vi "#SPI_TOF_LIDAR_cz_yuanshi.vi"() -> ()   [LabVIEW 2020]
uses:
  Control 1_.ctl
  Control 2_.ctl
  <vilib>/Analysis/baseanly.llb/Mean (DBL).vi
  handle_ALP_error.vi
  <vilib>/Utility/error.llb/Error Cluster From Error Code.vi
  <vilib>/Analysis/NI_AALBase.lvlib
  <vilib>/gmath/NI_Gmath.lvlib
panel:
  out "Rapid Block Acquisition Settings":T1={"preTriggerSamples"=0, "postTriggerSamples"=1000, "timebase"=2, "Four Channel Device"=FALSE, "Oversample"=1, "Number of Captures"=1}
  in  "index (row)":i32
  out "数组":i16[](array[numeric])
  in  "y 2":dbl
  in  "Tab Control 2":T2(tab)
  out "Resolution":i32=32 min=16 max=128 step=16
  in  "Max Resolution":enum16{"128", "64", "32", "16"}(ring)=enum."32"
  in  "Pulses/Pattern":i32=4
  in  "ms to wait":u32
  in  "Trigger Settings":T3={"Trigger Enabled"=TRUE, "Trigger Source"=enum."Channel C", "Trigger Threshold"=10, "Trigger Direction"=2, "Trigger Delay (samples)"=40, "Auto Trigger Time (ms)"=1000} {"Trigger Direction" items=["Rising"=2, "Falling"=3]}
  out "Captures":u32=10240
  in  "Post Trig. Samples":u32=30
  out "Patterns Loaded":dbl(slide)=2048.0 scale=0.0..2048.0
  in  "Initialised?":bool
  in  "y":dbl=0.9
  out "picture time s":dbl=0.0005142857142857143 format="%#.3p"
  out "1/x":dbl=0.00014285714285714287 format="%#.3p"
  in  "Pre Trigger Samples":u32
  in  "DMD Mode":enum16{"Slave - LUT", "Slave - All Patterns"}(ring)
  in  "Patterns to display":u32(slide)=1024 min=1 max=4096 step=1 scale=0.0..1024.0
  in  "Adaptive Slider":dbl(slide)=1.0 min=0.0 max=1.0 step=0.01 scale=0.0..1.0
  in  "Evolutionary":bool
  in  "Patterns":enum16{"Hadamard", "Random", "Democratised"}(ring)
  in  "learned":bool
  in  "Additional Data":dbl=1.25 format="%#_13g"
  in  "Smooth (pixels)":dbl=0.4 format="%#_13g"
  in  "ntimes":i32=4
  in  "Thresholded":bool
  in  "First":bool
  in  "upsample factor":i32=1
  in  "Depth Smooth":dbl=1.0 format="%#_13g"
  in  "depth threshold":dbl=1.0000000000000009
  in  "reflectivity threshold":dbl=0.35 format="%#_13g"
  out "updating":bool
  in  "fix":bool
  in  "Autofocus":bool
  in  "Height Scale":dbl=100.0 format="%#_13g"
  in  "max value":dbl=100.0 format="%#_13g"
  in  "min value":dbl format="%#_13g"
  in  "max reflectivity":dbl=1.0
  out "Update Rate (Hz)":dbl=45.45454545454545 format="%.2g"
  out "# elements 2":i32
  out "Total Rate (Hz)":dbl=45.45454545454545 format="%.2g"
  out "3D Display Rate (Hz)":dbl=111.11111111111111 format="%.2g"
  out "# elements 3":i32
  out "# elements":i32
  out "2D Rate (Hz)":dbl=inf format="%.2g"
  out "3D Rate (Hz)":dbl=inf format="%.2g"
  in  "Tab Control":T4(tab)=enum."Temporal Signals"
  out "?":dbl[](graph)
  out "?":dbl[](graph)
  out "pattern temporal signal":cluster{dbl[], dbl[]}(graph)
  out "?":dbl[](graph)
  out "OK?":bool
  in  "Save":bool
  in  "path":path=path "C:/Users/optics/Documents/Matt/Selex Partnership Project/Data/Lab Tests/Green/20160119/32 compressive/8 pulses"
  out "Depth + Reflectivity":T5
  out "Depth":T6
  out "Depth Map":dbl[][](graph)
  out "Reconstruction":dbl[][](graph)
  out "Hadamards":bool[][](array[boolean])
  in  "Channel A Settings":T7={"Enabled"=TRUE, "Coupling"=2, "Range"=3, "Analogue Offset"=0.0, "Bandwidth"=0} {"Bandwidth" items=["Full", "20 MHz"]; "Range" items=["10 mV", "20 mV", "50 mV", "100 mV", "200 mV", "500 mV", "1 V", "2 V", "5 V", "10 V", "20 V", "50 V ", "100 V"]; "Coupling" items=["AC", "DC 1 MOhm", "DC 50 Ohm"]}
  out "total patterns":i32=2048
  in  "Stop":bool=TRUE
  # "3000"
  # "maxADC=32512"
  # "400ps per delay point"
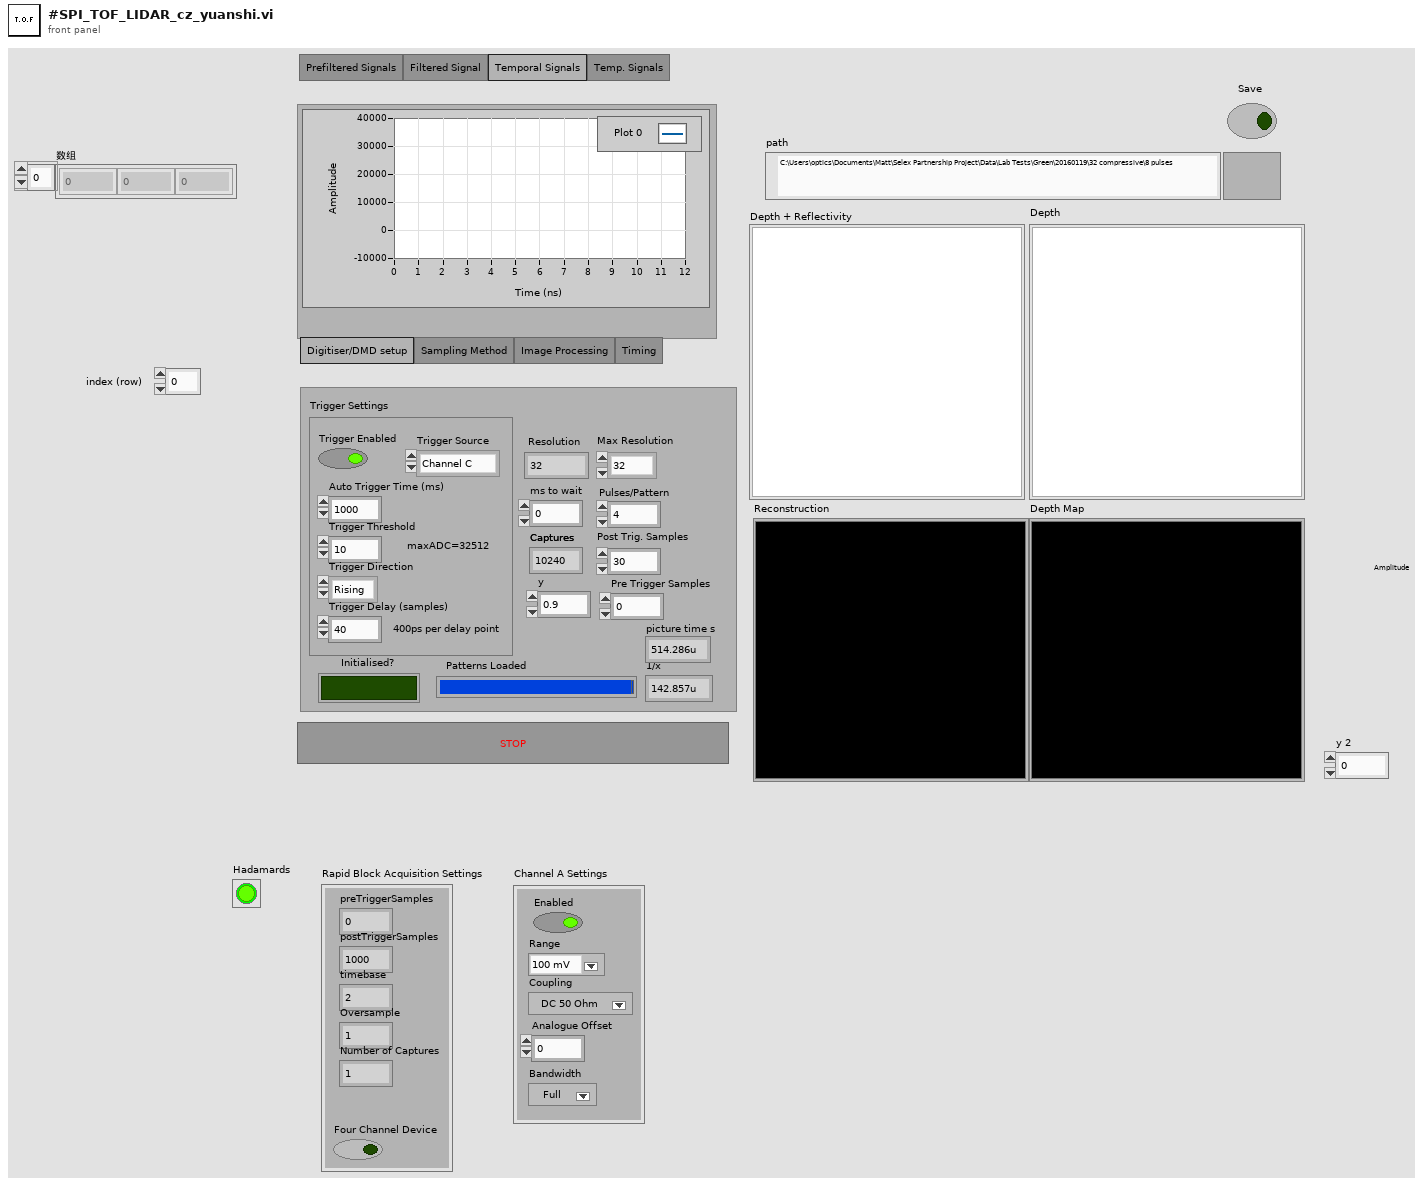
[diagram p1: front panel]
types:
  T1 = cluster{"preTriggerSamples":u32, "postTriggerSamples":u32, "timebase":u32, "Four Channel Device":bool, "Oversample":i16, "Number of Captures":u32}
  T2 = enum32{"Digitiser/DMD setup", "Sampling Method", "Image Processing", "Timing"}
  T3 = cluster{"Trigger Enabled":bool, "Trigger Source":enum32{"Channel A", "Channel B", "Channel C", "Channel D", "External", "Aux."}, "Trigger Threshold":i16, "Trigger Direction":u16, "Trigger Delay (samples)":u32, "Auto Trigger Time (ms)":i16}
  T4 = enum32{"Prefiltered Signals", "Filtered Signal", "Temporal Signals", "Temp. Signals"}
  T5 = typedef "Control 2_.ctl" = refnum<vi>
  T6 = typedef "Control 1_.ctl" = refnum<vi>
  T7 = cluster{"Enabled":bool, "Coupling":u32, "Range":u32, "Analogue Offset":sgl, "Bandwidth":u32}
  T8 = cluster{dbl[][], "All Patterns out":bool[][], "LUT":i32[]}
  T9 = typedef "imagedata.ctl" = cluster{"image type":i32, "image depth":i32, "image":u8[], "mask":u8[], "colors":u32[], "Rectangle":cluster{"left":i16, "top":i16, "right":i16, "bottom":i16}}
  T10 = cluster{"Pre Trigger Samples":u32, "Post Trig. Samples":u32, "timebase":u32, "Four Channel Device":bool, "Oversample":i16, u32}
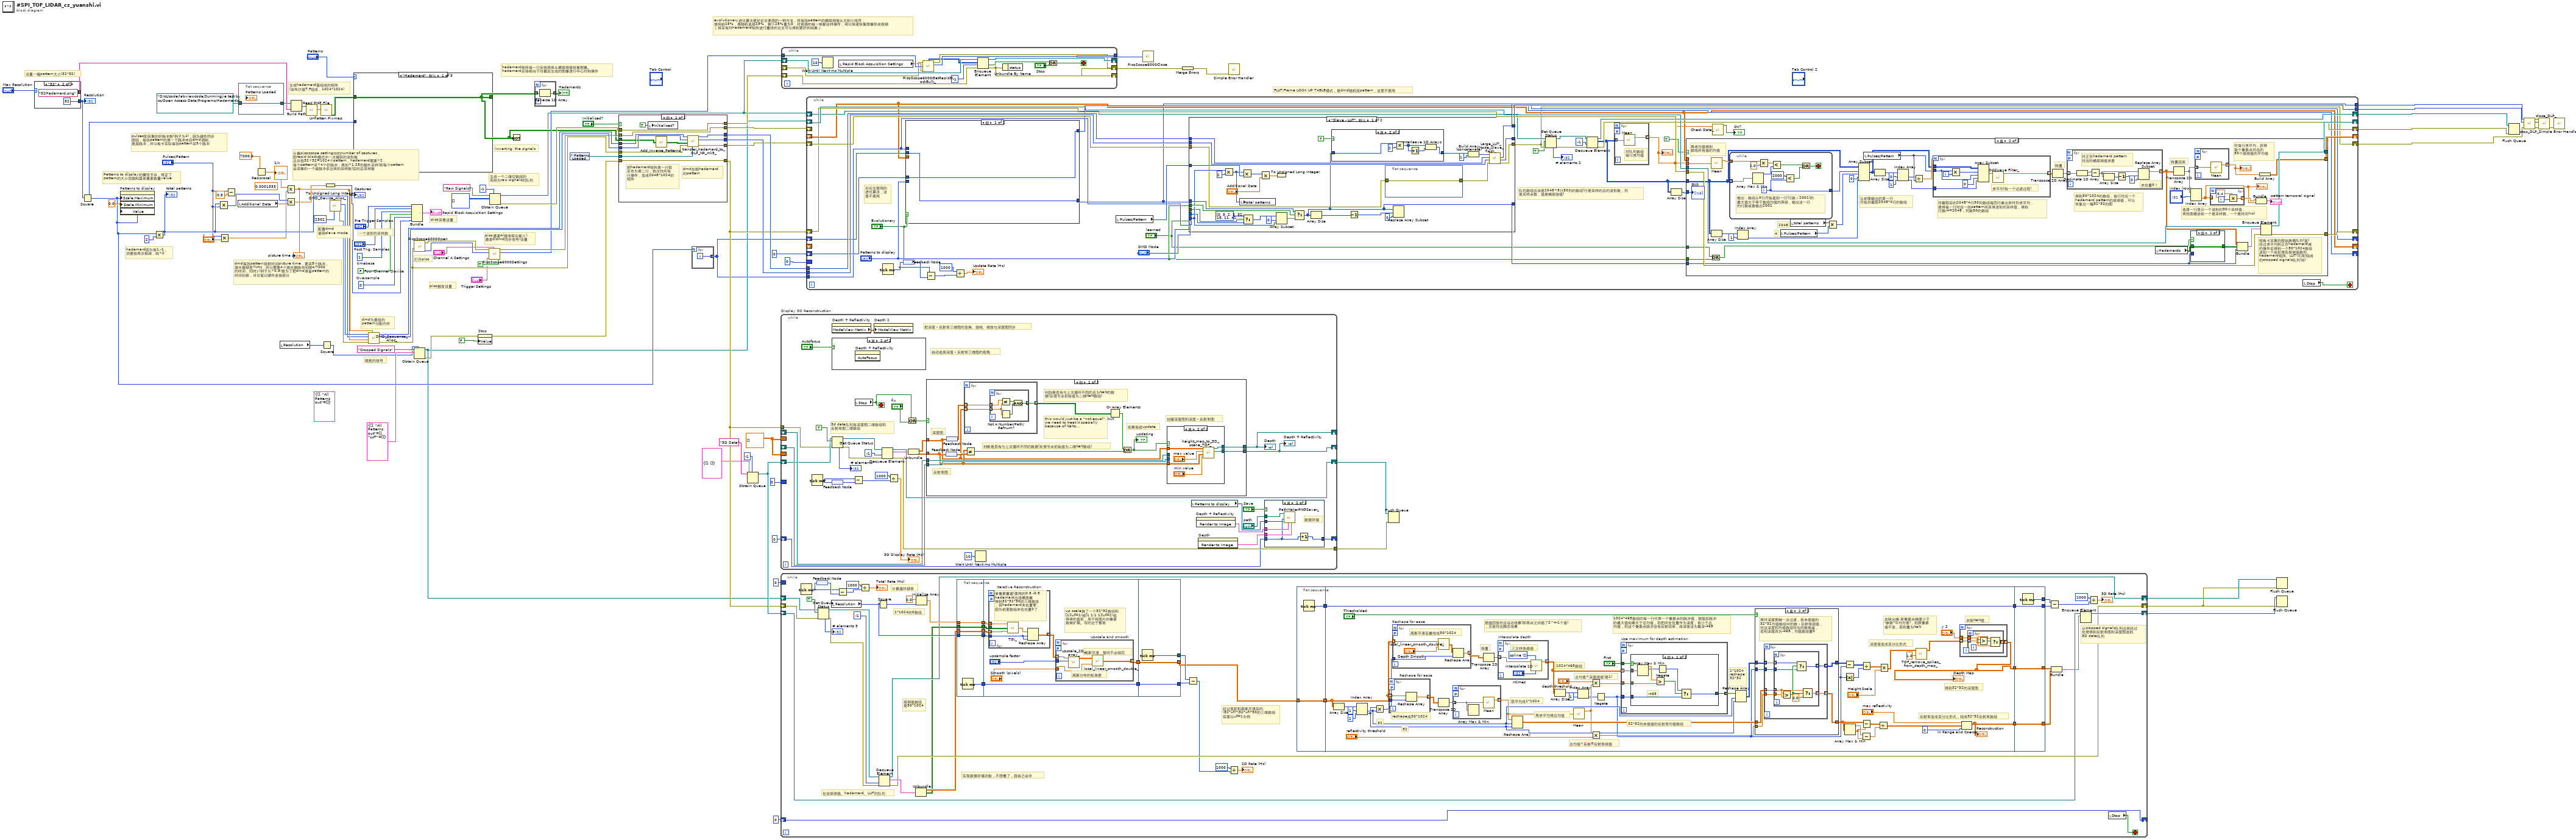
[diagram p0: block diagram]
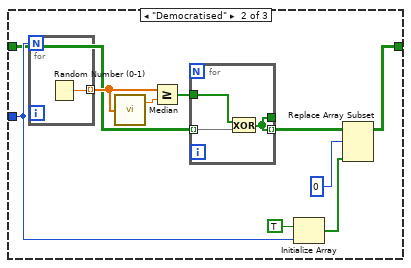
[diagram p2: hidden frame]
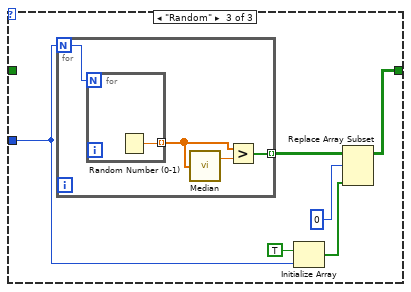
[diagram p3: hidden frame]
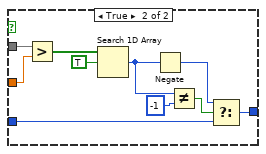
[diagram p9: hidden frame]
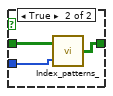
[diagram p11: hidden frame]
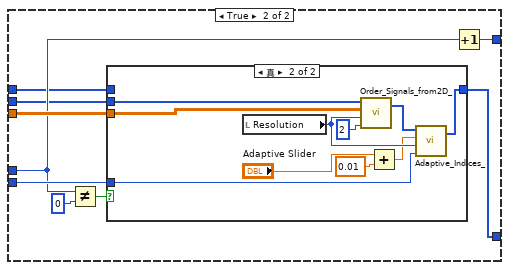
[diagram p12: hidden frame]
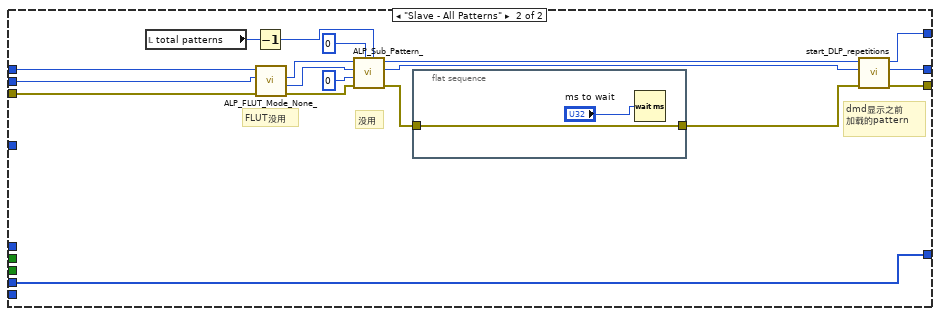
[diagram p15: hidden frame]
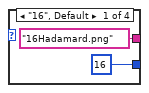
[diagram p17: hidden frame]
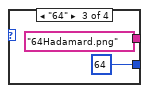
[diagram p18: hidden frame]
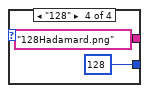
[diagram p19: hidden frame]
diagram:
  (unwired) cluster{dbl[][], "All Patterns out":bool[][]} {[], "All Patterns out"=[]} ("output cluster")
  w62 = dbl[][] [] ("Height Map")
  w6 = FALSE  # Four Channel Device
  w7 = u32 1  # timebase
  w3 = i16 0  # Oversample
  (unwired) 0.0001333 ("x")
  # "hadamard矩阵每一行反转用来从桶探测值恢复图像。\nhadamard反转相当于对最后生成的图像进行中心对称操作"
  # "pulses即采集的好脉冲数(例子为4)，因为硬件同步\n原因，每张pattern的第一个脉冲未经dmd调制，\n是废脉冲，所以板卡实际每张pattern采5个脉冲"
  # "裁剪的信号"
  # "evolutionary进化算法是孙论文使用的一种方法，将每张pattern的桶探测值从大到小排序，\n使用前25%，再随机选择25%，剩下25%置为0，对视频的每一帧都这样操作，用以快速恢复图像形成视频\n（其实有对hadamard矩阵进行重排的论文可以得到更好的结果）"
  # "生成一个二维空数组的\n名称为raw signals的队列"
  # "FLUT:Frame LOOK UP TABLE模式，是dmd随机投pattern，这里不使用"
  # "pico采集设置"
  # "pico通道A(接收探头输入).\n通道C(dmd同步信号)设置"
  # "pico触发设置"
  # "打开pico"
  # "配置dmd\n使用slave mode"
  # "dmd为要投的\npattern分配内存"
  # "dmd每张pattern投射时间picture time，要采5个脉冲，\n激光器频率7kHz，所以需要4个激光器脉冲间隔4/7000\n的时间，同时y(例子为×0.9)是为了把dmd准备pattern的\n时间扣掉，详见笔记硬件连接部分"
  # "一个波形的采样数"
  # "计算picoscope setting中的number of captures，\n即rapid block模式中一次捕获的波形数\n总共投32×32=1024个pattern，hadamard需要×2，\n每个pattern采×4个好脉冲，再加×1.25的额外采样(即每个pattern\n会采集的一个废脉冲多出来的采样数)后的总采样数"
  # "hadamard因为有1.-1，\n须要投两次相减，故×2"
  # "Patterns to display的属性节点，规定了\npattern的大小范围和具体像素数量value"
  # "生成hadamard基组成的矩阵\n(由布尔值T.F组成，1024*1024)"
  # "设置一幅pattern大小(32*32)"
  # "inverting  the signals"
  n1 = case shown="\"32\"" "Max Resolution" {
    tunnel: [16 32 64 128] -> w40
    tunnel: ["16Hadamard.png" ("string") "32Hadamard.png" ("string") "64Hadamard.png" ("string") "128Hadamard.png" ("string")] -> w22
    frame "16", Default {
    }
    frame "32" {
    }
    frame "64" {
    }
    frame "128" {
    }
  }
  "Resolution" <- w40
  n2 = Square(x=w40) -> (x^2=w38:i32)
  n3 = property on="Patterns to display" class="Slide (严格)"("Scale.Maximum"=w38, "Scale.Minimum"=0.0 ("Scale.Range:Minimum"), "Value"=w38) -> ()  [unwired: 2 in, 2 out]
  n4 = Multiply(x=w38, y=2) -> (x*y=w39:i32)
  "total patterns" <- w39
  n5 = Multiply(x=w39, y="Pulses/Pattern") -> (x*y=w67:i32)
  n6 = Multiply(x="Pulses/Pattern", y="y") -> (x*y=w18:dbl)
  n7 = Subtract(x="Pulses/Pattern", y=0.5) -> ()  [unwired: 1 out]
  n8 = local read "Additional Data"() -> (w43:dbl)
  n9 = flat-sequence {
    tunnel: path "D:/cz/code/labviewcode/Sunmingjie test by cz/Open Access Data/Programs/Hadamards" ("Folder to Store Files 2") -> [w104]
    tunnel: [w104] -> w23
    frame #0 {
    }
  }
  n10 = Reciprocal(x=7000.0 ("laser rep rate")) -> (1/x=w15:dbl)
  "1/x" <- w15
  n11 = local read "Resolution"() -> (w65:i32)
  n12 = Multiply(x=w15, y=w18) -> (x*y=w89:dbl)
  "picture time s" <- w89
  n13 = Multiply(x=w67, y=w43) -> (x*y=w73:dbl)
  n14 = Build Path(base path=w23, name or relative path=w22) -> (appended path=w21:path)
  n15 = call <vilib>:"Read PNG File.vi"("path to PNG file"=w21) -> ("image data"=w25:T9)  [unwired: 8 in, 2 out]
  n16 = call <vilib>:"Unflatten Pixmap.vi"("image data"=w25) -> ("1-bit pixmap"=w24:bool[][])  [unwired: 4 in, 6 out]
  n17 = Square(x=w65) -> (x^2=w12:i32)
  n18 = To Unsigned Long Integer(number=w73) -> (unsigned 32bit integer=w2:u32)
  "Captures" <- w2
  n19 = call "DMD_Device_Alloc_.vi"("Master/Slave Mode"=2302) -> ("error out"=w94:errorcluster, "DeviceIdPtr"=w95:u32)  [unwired: 8 in, 1 out]
  n20 = case shown="\"Hadamard\", 默认" "Patterns" {
    tunnel: w38 -> [_ w115 w121]
    tunnel: [w105 w111 w120] -> w14
    tunnel: w24 -> [w105 w109 _]
    frame "Hadamard", Default {
    }
    frame "Democratised" {
      n21 = for {
        N: w115 -> [_]
        tunnel: [w119] -> w110 mode=indexing
        n22 = Random Number (0-1)() -> (number: 0 to 1=w119:dbl)
      }
      n23 = call <vilib>:"Median.vi"("X"=w110) -> ("median"=w107:dbl)  [unwired: 1 out]
      n24 = Greater Or Equal?(x=w110, y=w107) -> (x >= y?=w106:bool[])
      n25 = for {
        tunnel: w106 -> [w118]
        tunnel: w109 -> [w117] mode=indexing
        tunnel: [w116] -> w108 mode=indexing
        tunnel: [w116] -> _
        n26 = Exclusive Or(1:w117, 2:w118) -> (0:w116:bool[])
      }
      n27 = Initialize Array(TRUE, w115) -> (w113:bool[])
      n28 = Replace Array Subset(array=w108, new element=w113, index (row)=0) -> (w111:bool[][])  [unwired: 1 in]
    }
    frame "Random" {
      n29 = for {
        N: w121 -> [w129]
        tunnel: [w126] -> w123 mode=indexing
        n30 = for {
          N: w129 -> [_]
          tunnel: [w130] -> w127 mode=indexing
          n31 = Random Number (0-1)() -> (number: 0 to 1=w130:dbl)
        }
        n32 = call <vilib>:"Median.vi"("X"=w127) -> ("median"=w128:dbl)  [unwired: 1 out]
        n33 = Greater?(x=w127, y=w128) -> (0:w126:bool[])
      }
      n34 = Initialize Array(TRUE, w121) -> (w124:bool[])
      n35 = Replace Array Subset(array=w123, new element=w124, index (row)=0) -> (w120:bool[][])  [unwired: 1 in]
    }
  }
  n36 = call "DMD_Sequence_Alloc_.vi"("Picture Time (s)"=w89, "error in (no error)"=w94, "Illuminate Time (s)"=w89, "Number of Frames"=w39, "DeviceIdPtr in"=w95) -> ("error out"=w42:errorcluster, "SequenceId"=w86:u32, "DeviceIdPtr out"=w87:u32)  [unwired: 3 in, 1 out]
  n37 = Bundle("Pre Trigger Samples"="Pre Trigger Samples", "Post Trig. Samples"="Post Trig. Samples", "timebase"=w7, "Four Channel Device"=w6, "Oversample"=w3, w2) -> (→"Rapid Block Acquisition Settings":T10)  [unwired: 1 in]
  n38 = call "PicoScope6000Open.vi"("error in (no error)"=w42) -> ("handle"=w75:i16, "error out"=w76:errorcluster)  [unwired: 2 in, 2 out]
  n39 = Obtain Queue(max queue size (-1, unlimited)=w12, name (unnamed)="Cropped Signals", element data type=T8 {[], "All Patterns out"=[], "LUT"=[]} ("output cluster")) -> (queue out=w10:refnum<queue>, error out=w46:errorcluster)  [unwired: 2 in, 1 out]
  n40 = property on="Stop" class="Bool (严格)"(error in=w46, "Value"=FALSE ("Stop")) -> (error out=w45:errorcluster)  [unwired: 1 in, 1 out]
  n41 = call "PicoScope6000Settings.vi"("PS6407?"=TRUE, "Channel A Settings"="Channel A Settings", "Trigger Settings"="Trigger Settings", "handle in"=w75, "error in"=w76) -> ("handle out"=w51:i16, "error out"=w54:errorcluster)  [unwired: 4 in, 1 out]
  n42 = Obtain Queue(max queue size (-1, unlimited)=-1, name (unnamed)="Raw Signals", element data type=i16[][] [] ("Channel A Buffer")) -> (queue out=w11:refnum<queue>, error out=w53:errorcluster)  [unwired: 2 in, 1 out]
  n43 = Not(x=w14) -> ()  [unwired: 1 out]
  n44 = for {
    tunnel: w14 -> [w132] mode=indexing
    tunnel: [w131] -> w13 mode=indexing
    n45 = Reverse 1D Array(array=w132) -> (reversed array=w131:bool[])
  }
  "Hadamards" <- w13
  n46 = control-ref of="Patterns Loaded"() -> (w82:refnum<vi>)
  n47 = case shown="假" "Initialised?" {
    tunnel: w87 -> [w144 w151]
    tunnel: w42 -> [w143 w150]
    tunnel: [w140 w151] -> w85
    tunnel: [w139 w149] -> w84
    tunnel: [w141 w150] -> w68
    tunnel: w82 -> [w142 _]
    tunnel: w86 -> [w138 w149]
    tunnel: w14 -> [w137 _]
    tunnel: [w135 w148] -> w49
    tunnel: w54 -> [w135 w148]
    tunnel: [w134 w147] -> w52
    tunnel: w53 -> [w134 w147]
    tunnel: w45 -> [w133 w146]
    tunnel: [w133 w146] -> w44
    frame False {
      # "dmd加载hadamard\n的pattern"
      # "把hadamard矩阵第一行取\n反作为第二行，依次对所有\n行操作，变成2048*1024的\n矩阵"
      n48 = local write "Initialised?"(TRUE ("Initialised?")) -> ()
      n49 = call "Add_Inverse_Patterns_.vi"("Hadamard"=w137) -> ("Array"=w136:bool[][])
      n50 = call "transfer_hadamard_to_DLP_NR_mk3_.vi"("Progress Indicator"=w142, "error in (no error)"=w143, "Hadamard"=w136, "SequenceId"=w138, "DeviceId"=w144) -> ("error out"=w141:errorcluster, "SequenceId Out"=w139:u32, "DeviceId Out"=w140:u32)  [unwired: 4 in]
    }
    frame True {
    }
  }
  n51 = for {
    N: w38 -> [_]
    tunnel: [w152] -> w41 mode=indexing
    i -> [w152]
  }
  n52 = Obtain Queue(max queue size (-1, unlimited)=-1, name (unnamed)="3D Data", element data type=cluster{dbl[][], dbl[][]} {[], []} ("3D Data")) -> (queue out=w57:refnum<queue>)  [unwired: 2 in, 2 out]
  n53 = while {
    shift-right: [w197] -> w33
    shift-left: w10 -> [w183]
    shift-right: [w196] -> w34
    shift-left: w57 -> [w195]
    shift-right: [w192] -> w32
    shift-left: w44 -> [w182]
    border: u32 0 ("millisecond timer value") -> [_]
    shift-right: [w153] -> _
    shift-left: u32 0 ("millisecond timer value") -> [w153]
    stop <- w199 stop-if-true
    # "从cropped signals队列出来经过\n处理得到反射率图和深度图送到\n3D data队列"
    # "经过直积和高斯平滑后的\n(32*uf)*(32*uf)*30的三维数组\n后面以uf=1为例"
    # "探测值数组\n是30*1024"
    # "包含探测值、hadamard、LUT的队列"
    # "1*1024的0数组"
    # "计算循环频率"
    # "实现数据存储功能，不想看了，我自己会存"
    n54 = Tick Count (ms)() -> (millisecond timer value=w188:u32)
    n55 = feedback #1() -> (w189:u32)
    n56 = feedback-in #1(w188) -> ()
    n57 = Get Queue Status(queue=w183, return elements? (F)=TRUE, error in (no error)=w182) -> (queue out=w181:refnum<queue>, error out=w180:errorcluster, # elements in queue=→"# elements 3":i32)  [unwired: 5 out]
    n58 = local read "Resolution"() -> (w198:i32)
    n59 = Subtract(x=w188, y=w189) -> (x-y=w187:u32)
    n60 = Divide(x=u32 1000, y=w187) -> (x/y=→"Total Rate (Hz)":dbl)
    n61 = Square(x=w198) -> (x^2=w203:i32)
    n62 = Dequeue Element(queue=w181, timeout in ms (-1)=-1, error in (no error)=w180) -> (queue out=w197:refnum<queue>, element=w193:T8, error out=w192:errorcluster)  [unwired: 1 out]
    n63 = Unbundle(w193) -> (w155:dbl[][], "All Patterns out"=w154:bool[][])  [unwired: 1 out]
    n64 = Initialize Array(0.0 ("element"), w203) -> (w201:dbl[])
    n65 = flat-sequence {
      tunnel: w154 -> [w324]
      tunnel: w155 -> [w325]
      tunnel: w198 -> [w326]
      tunnel: w201 -> [w327]
      tunnel: [w327] -> w178
      tunnel: [w326] -> w177
      tunnel: [w325] -> w176
      tunnel: [w324] -> w175
      tunnel: [w323] -> w168
      tunnel: w178 -> [w336]
      tunnel: w177 -> [w335]
      tunnel: w176 -> [w333]
      tunnel: w175 -> [w332]
      tunnel: [w329] -> w174
      tunnel: w168 -> [w328]
      tunnel: [w328] -> w167
      tunnel: [w350] -> w166
      tunnel: w174 -> [w350]
      tunnel: [w349] -> w170
      tunnel: [w348] -> w169
      tunnel: w167 -> [w348]
      frame #0 {
        n66 = Tick Count (ms)() -> (millisecond timer value=w323:u32)
      }
      frame #1 {
        # "up scale做了一个32*32数组和\n[1](uf=1)或[1 1;1 1](uf=2)或\n等等的直积，用于将图片的像素\n数做扩展。写的过于繁琐"
        n67 = for "Iterative Reconstruction" {
          tunnel: w333 -> [w343] mode=indexing
          tunnel: w335 -> [w347]
          tunnel: [w345] -> w331 mode=indexing
          tunnel: w336 -> [w346]
          tunnel: w332 -> [w344]
          workers-P: _ -> [_]
          # "单像素重建(使用的0.5,-0.5\nhadamard出场景图像\n得到32*32*30的三维数组\n，但hadamard末位置零，\n因为前面数组末位也置0了"
          n68 = call "TGI_.vi"("Signals"=w343, "Hadamard"=w344, "Initialise Array"=w346) -> ("Reconstruction"=w342:dbl[])
          n69 = Reshape Array(w342, w347, w347) -> (w345:dbl[][])
        }
        n70 = for "Upscale and smooth" {
          tunnel: w331 -> [w341] mode=indexing
          tunnel: "Smooth (pixels)" -> [w340]
          tunnel: [w338] -> w329 mode=indexing
          tunnel: "upsample factor" -> [w337]
          workers-P: _ -> [_]
          # "高斯分布的标准差"
          # "高斯平滑，暂时不必细究"
          n71 = call "Upscale_2D_array_.vi"("Upsample Factor"=w337, "Small Array"=w341) -> ("Big Array"=w339:dbl[][])  [unwired: 7 in, 2 out]
          n72 = call "local_linear_smooth_double_.vi"("Smoothing Parameter (Gaussian S.D. in pixels)"=w340, "Input Array"=w339) -> ("Smoothed Array"=w338:dbl[][])
        }
      }
      frame #2 {
        n73 = Tick Count (ms)() -> (millisecond timer value=w349:u32)
      }
    }
    n74 = Subtract(x=w170, y=w169) -> (x-y=w171:u32)
    n75 = Divide(x=u32 1000, y=w171) -> (x/y=→"2D Rate (Hz)":dbl)
    n76 = flat-sequence {
      tunnel: w166 -> [w205]
      tunnel: [w205] -> w165
      tunnel: [w204] -> w158
      tunnel: w165 -> [w211]
      tunnel: [w213] -> w164
      tunnel: [w209] -> w163
      tunnel: [w235] -> w159
      tunnel: w158 -> [w235]
      tunnel: [w321] -> w190
      tunnel: [w322] -> w191
      tunnel: w164 -> [w322]
      tunnel: w163 -> [w321]
      tunnel: [w320] -> w157
      tunnel: w159 -> [w320]
      tunnel: [w319] -> w156
      frame #0 {
        n77 = Tick Count (ms)() -> (millisecond timer value=w204:u32)
      }
      frame #1 {
        # "去除尖峰,若像素点梯度小于\n(参数*平均方差)，则原像素\n值不变，否则置为NaN"
        # "得到32*32的深度图"
        # "去除NaN值"
        # "反射率变成百分比形式，组成32*32反射率数组"
        # "深度值变成百分比形式"
        # "1*1024\nreshape\n32*32"
        # "32"
        # "32"
        # "reshape成30*1024"
        # "1024*465数组的每一行代表一个像素点的脉冲值，插值后脉冲\n的最大值如果大于总均值，则把所在位置作为深度，若小于总\n均值，则这个像素点脉冲没有反射回来，故深度设为最深-465"
        # "1024*465数组"
        # "转置"
        # "32*32的未插值的反射率均值数组"
        # "总均值×深度阈值(是1)"
        # "总均值×系数=反射率阈值"
        # "再求平均得总均值"
        # "取平均成1*1024"
        # "插值四倍对应运动场景(即两点之间插了2^4-1个值)\n，五倍对应静态场景"
        n78 = Array Size(array=w211) -> (size(s)=w252:i32[])
        n79 = Index Array(array=w252, index #1=1 ("index"), index #2=2 ("index")) -> (element #1=w246:i32, element #2=w245:i32)
        n80 = Multiply(x=w245, y=w246) -> (x*y=w239:i32)
        n81 = for "Reshape for ease" {
          tunnel: w211 -> [w314] mode=indexing
          tunnel: w239 -> [w313]
          tunnel: [w312] -> w249 mode=indexing
          workers-P: _ -> [_]
          n82 = Reshape Array(w314, w313) -> (w312:dbl[])
        }
        n83 = for "Reshape for ease" {
          tunnel: w239 -> [w260]
          tunnel: [w264] -> w237 mode=indexing
          tunnel: w211 -> [w263] mode=indexing
          workers-P: _ -> [_]
          # "高斯平滑后重排成30*1024"
          n84 = call "local_linear_smooth_double_.vi"("Smoothing Parameter (Gaussian S.D. in pixels)"="Depth Smooth", "Input Array"=w263) -> ("Smoothed Array"=w262:dbl[][])
          n85 = Reshape Array(w262, w260) -> (w264:dbl[])
        }
        n86 = Transpose 2D Array(2D array=w249) -> (transposed array=w248:dbl[][])
        n87 = for {
          tunnel: w248 -> [w288] mode=indexing
          tunnel: [w287] -> w247 mode=indexing
          workers-P: _ -> [_]
          n88 = Array Max & Min(array=w288) -> ()  [unwired: 4 out]
          n89 = call-poly <vilib>:"Mean.vi"("X"=w288) -> ("mean"=w287:dbl)  [unwired: 1 out]
        }
        n90 = Transpose 2D Array(2D array=w237) -> (transposed array=w238:dbl[][])
        n91 = for "Interpolate depth" {
          tunnel: w238 -> [w318] mode=indexing
          tunnel: [w316] -> w234 mode=indexing
          workers-P: _ -> [_]
          w317 = 2 items=["nearest", "linear", "spline", "cubic Hermite", "Lagrange"] ("method")
          # "三次样条插值"
          n92 = call <vilib>:"Interpolate 1D.vi"("ntimes"="ntimes", "method"=w317, "Y"=w318) -> ("yi"=w316:dbl[])  [unwired: 6 in, 2 out]
        }
        n93 = Reshape Array(w247, w246, w245) -> (w243:dbl[][])
        n94 = Array Size(array=w234) -> (size(s)=w233:i32[])
        n95 = call-poly <vilib>:"Mean.vi"("X"=w247) -> ("mean"=w230:dbl)  [unwired: 1 out]
        n96 = Index Array(array=w233, index=1) -> (element=w220:i32)
        n97 = Multiply(x="depth threshold", y=w230) -> (x*y=w241:dbl)
        n98 = Multiply(x=w230, y="reflectivity threshold") -> (x*y=w228:dbl)
        n99 = Negate(x=w220) -> (-x=w227:i32)
        n100 = for "Use maximum for depth estimation" {
          tunnel: w234 -> [w290] mode=indexing
          tunnel: [w292] -> w236 mode=indexing
          tunnel: w241 -> [w293]
          workers-P: _ -> [_]
          tunnel: w227 -> [w291]
          tunnel: "First" -> [w289]
          n101 = case shown="假" w289 {
            tunnel: w293 -> [w299 w311]
            tunnel: [w294 w305] -> w292
            tunnel: w291 -> [w295 w303]
            tunnel: w290 -> [w301 w302]
            frame False {
              # "-465"
              n102 = Array Max & Min(array=w301) -> (max value=w300:dbl, max index (indices)=w297:i32)  [unwired: 2 out]
              n103 = Greater?(x=w300, y=w299) -> (0:w296:bool)
              n104 = Negate(x=w297) -> (-x=w298:i32)
              n105 = Select(t=w298, s=w296, f=w295) -> (s? t:f=w294:i32)
            }
            frame True {
              n106 = Greater?(x=w302, y=w311) -> (0:w310:bool[])
              n107 = Search 1D Array(1D array=w310, element=TRUE) -> (index of element=w304:i32)  [unwired: 1 in]
              n108 = Negate(x=w304) -> (-x=w306:i32)
              n109 = Not Equal?(x=w304, y=-1) -> (x != y?=w307:bool)
              n110 = Select(t=w306, s=w307, f=w303) -> (s? t:f=w305:i32)
            }
          }
        }
        n111 = Reshape Array(w236, w246, w245) -> (w242:i32[][])
        n112 = case shown="真" "Thresholded" {
          tunnel: w243 -> [w266 w271]
          tunnel: w228 -> [_ w272]
          tunnel: [w266 w267] -> w222
          tunnel: w242 -> [w265 w270]
          tunnel: [w265 w268] -> w212
          tunnel: w227 -> [_ w269]
          frame False {
          }
          frame True {
            # "再对深度图做一次过滤，若未插值的\n32*32均值数组中的数＞反射率阈值，\n对应深度和均值数组对应的数保留，\n否则深度改为-465，均值数组置0"
            n113 = for {
              tunnel: [w278] -> w267 mode=indexing
              tunnel: w271 -> [w277] mode=indexing
              tunnel: w272 -> [w276]
              tunnel: w270 -> [w275] mode=indexing
              tunnel: w269 -> [w273]
              tunnel: [w274] -> w268 mode=indexing
              n114 = for {
                tunnel: [w286] -> w278 mode=indexing
                tunnel: w277 -> [w284] mode=indexing
                tunnel: w276 -> [w285]
                tunnel: w275 -> [w281] mode=indexing
                tunnel: w273 -> [w280]
                tunnel: [w279] -> w274 mode=indexing
                n115 = Greater?(x=w284, y=w285) -> (0:w282:bool)
                n116 = Select(t=w281, s=w282, f=w280) -> (s? t:f=w279:i32)
                n117 = Select(t=w284, s=w282, f=0.0) -> (s? t:f=w286:dbl)
              }
            }
          }
        }
        n118 = Subtract(x=w212, y=w227) -> (x-y=w221:i32[][])
        n119 = Absolute Value(x=w227) -> (abs(x)=w218:i32)
        n120 = Array Max & Min(array=w222) -> (max value=w226:dbl, min value=w225:dbl)  [unwired: 2 out]
        n121 = Subtract(x=w226, y=w225) -> (x-y=w223:dbl)
        n122 = Divide(x=w221, y=w218) -> (x/y=w219:dbl[][])
        n123 = Subtract(x=w222, y=w225) -> (x-y=w224:dbl[][])
        n124 = Divide(x=w224, y=w223) -> (x/y=w216:dbl[][])
        n125 = Multiply(x=w219, y="Height Scale") -> (x*y=w208:dbl[][])
        n126 = call "TOF_remove_spikes_from_depth_map_.vi"("threshold for spike removal (standard deviations)"=1.0, "Depth Map"=w208) -> ("Depth Map (no spikes)"=w207:dbl[][])  [unwired: 9 in]
        n127 = for {
          tunnel: [w255] -> w209 mode=indexing
          tunnel: w207 -> [w254] mode=indexing
          tunnel: "y 2" -> [w253]
          n128 = for {
            tunnel: [w258] -> w255 mode=indexing
            tunnel: w254 -> [w257] mode=indexing
            tunnel: w253 -> [w256]
            n129 = Greater?(x=w257, y=w256) -> (0:w259:bool)
            n130 = Select(t=w257, s=w259, f=w256) -> (s? t:f=w258:dbl)
          }
        }
        "Depth Map" <- w209
        n131 = In Range and Coerce(upper limit="max reflectivity", x=w216, lower limit=0 ("index (row)")) -> (coerced(x)=w213:dbl[][])  [unwired: 1 out]
        "Reconstruction" <- w213
      }
      frame #2 {
        n132 = Tick Count (ms)() -> (millisecond timer value=w319:u32)
      }
    }
    n133 = Subtract(x=w156, y=w157) -> (x-y=w160:u32)
    n134 = Bundle(w190, w191) -> (w194:cluster{dbl[][], dbl[][]})  [unwired: 1 in]
    n135 = Enqueue Element(queue=w195, element=w194) -> (queue out=w196:refnum<queue>)  [unwired: 2 in, 2 out]
    n136 = Divide(x=u32 1000, y=w160) -> (x/y=→"3D Rate (Hz)":dbl)
    n137 = local read "Stop"() -> (w199:bool)
  }
  n138 = while "Display 3D Reconstruction" {
    shift-right: [w359] -> _
    shift-left: _ -> [w384]
    shift-right: [w358] -> _
    shift-left: _ -> [w383]
    border: w62 -> [_]
    border: w62 -> [_]
    shift-right: [w379] -> w61
    shift-left: w57 -> [w363]
    tunnel: w44 -> [w361]
    tunnel: [w371] -> w50
    border: u32 0 ("millisecond timer value") -> [_]
    shift-right: [w354] -> _
    shift-left: u32 0 ("millisecond timer value") -> [w355]
    stop <- w372 stop-if-true
    # "自动选择深度＋反射率三维图的视角"
    # "把深度＋反射率三维图的变换、旋转、缩放与深度图同步"
    # "3d data队列有深度图二维数组和\n反射率图二维数组"
    n139 = Tick Count (ms)() -> (millisecond timer value=w369:u32)
    n140 = case shown="真" "Autofocus" {
      frame False {
      }
      frame True {
        n141 = invoke on="Depth + Reflectivity" class="SceneGraphDisp (strict)" method="AutoFocus"() -> ()  [unwired: 3 in, 3 out]
      }
    }
    n142 = Get Queue Status(queue=w363, return elements? (F)=TRUE, error in (no error)=w361) -> (queue out=w362:refnum<queue>, error out=w360:errorcluster, # elements in queue=→"# elements":i32)  [unwired: 5 out]
    n143 = feedback #2() -> (w370:u32)
    n144 = feedback-in #2(w369) -> ()
    n145 = property on="Depth + Reflectivity" class="SceneGraphDisp (严格)"() -> ("ModelView Matrix"=w382:sgl[][])  [unwired: 2 in, 2 out]
    n146 = Subtract(x=w369, y=w370) -> (x-y=w368:u32)
    n147 = local read "Stop"() -> (w372:bool)
    n148 = property on="Depth 2" class="SceneGraphDisp (严格)"("ModelView Matrix"=w382) -> ()  [unwired: 2 in, 2 out]
    n149 = Dequeue Element(queue=w362, timeout in ms (-1)=-1, error in (no error)=w360) -> (queue out=w379:refnum<queue>, element=w378:cluster{dbl[][], dbl[][]}, error out=w371:errorcluster)  [unwired: 1 out]
    n150 = Divide(x=u32 1000, y=w368) -> (x/y=→"3D Display Rate (Hz)":dbl)
    n151 = Or(x=w372, y="fix") -> (x .or. y?=w373:bool)
    n152 = Unbundle(w378) -> (w376:dbl[][], w377:dbl[][])
    n153 = case shown="假" w373 {
      tunnel: w384 -> [w402 w421]
      tunnel: w383 -> [w401 w420]
      tunnel: [w400 w420] -> w358
      tunnel: [w399 w421] -> w359
      tunnel: w377 -> [w394 _]
      tunnel: w376 -> [w392 _]
      frame False {
        # "如果有就update"
        # "创建深度图和深度＋反射率图"
        # "判断是否有与上次循环不同的数据(反馈节点初始值为二维NaN数组)"
        # "判别是否有与上次循环不同的且为NaN的数\n据(反馈节点初始值为二维NaN数组)"
        # "反射率图"
        # "深度图"
        # "this would just be a \"not equal\", but we need to treat it specially because of NaNs..."
        n154 = feedback #3() -> (w403:dbl[][])
        n155 = feedback-in #3(w394) -> ()
        n156 = feedback #4() -> (w397:dbl[][])
        n157 = feedback-in #4(w392) -> ()
        n158 = for {
          tunnel: w397 -> [w406] mode=indexing
          tunnel: w392 -> [w405] mode=indexing
          tunnel: [w404] -> w396 mode=indexing
          n159 = for {
            tunnel: w406 -> [w411] mode=indexing
            tunnel: w405 -> [w410] mode=indexing
            tunnel: [w407] -> w404 mode=indexing
            n160 = Not Equal?(x=w411, y=w410) -> (x != y?=w408:bool)
            n161 = Not A Number/Path/Refnum?(number/path/refnum=w410) -> (NaN/Path/Refnum?=w409:bool)
            n162 = Compound Arithmetic op=AND(w408, invert w409) -> (w407:bool)
          }
        }
        n163 = Not Equal?(x=w394, y=w403) -> (x != y?=w398:bool)
        n164 = Or Array Elements(Boolean array=w396) -> (logical OR=w395:bool)
        n165 = Or(x=w395, y=w398) -> (x .or. y?=w393:bool)
        "updating" <- w393
        n166 = case shown="真" w393 {
          tunnel: [w413 w417] -> w399
          tunnel: [w412 w416] -> w400
          tunnel: w392 -> [_ w419]
          tunnel: w394 -> [_ w418]
          tunnel: w402 -> [w413 _]
          tunnel: w401 -> [w412 _]
          frame False {
          }
          frame True {
            n167 = call "height_map_to_3D_scene_TOF_.vi"("min value"="min value", "Reflectivity"=w418, "max value"="max value", "Height Map"=w419) -> ("3D Scene (textured)"=w416:refnum<vi>, "3D Scene (height map)"=w417:refnum<vi>)  [unwired: 1 in, 2 out]
          }
        }
      }
      frame True {
      }
    }
    "Depth + Reflectivity" <- w358
    "Depth" <- w359
    n168 = Wait Until Next ms Multiple(millisecond multiple=u32 10) -> ()  [unwired: 1 out]
    n169 = local read "Patterns to display"() -> (w352:u32)
    n170 = invoke on="Depth + Reflectivity" class="SceneGraphDisp (strict)" method="Render to Image"() -> ("Get Image"=w353:T9)  [unwired: 3 in, 2 out]
    n171 = invoke on="Depth" class="SceneGraphDisp (strict)" method="Render to Image"() -> ("Get Image"=w356:T9)  [unwired: 3 in, 2 out]
    n172 = case shown="真" "Save" {
      tunnel: w356 -> [_ w389]
      tunnel: w353 -> [_ w390]
      tunnel: w355 -> [w385 w388]
      tunnel: [w385 w391] -> w354
      tunnel: w352 -> [_ w387]
      tunnel: "path" -> [_ w386]
      frame False {
      }
      frame True {
        # "数据存储"
        n173 = call "PathMakerPNGSaver_.vi"("Height"=w389, "Reflectivity"=w390, "patterns"=w387, "frame number"=w388, "path"=w386) -> ()  [unwired: 5 in, 2 out]
        n174 = Increment(x=w388) -> (x+1=w391:u32)
      }
    }
  }
  n175 = while {
    shift-right: [w434] -> _
    shift-left: w11 -> [w435]
    tunnel: w51 -> [w433]
    shift-right: [w429] -> _
    shift-left: _ -> [w428]
    shift-right: [w427] -> w70
    shift-left: w52 -> [w430]
    tunnel: [w425] -> w69
    stop <- w426 stop-if-true
    n176 = Wait Until Next ms Multiple(millisecond multiple=u32 10) -> ()  [unwired: 1 out]
    n177 = local read "Rapid Block Acquisition Settings"() -> (w422:T1)
    n178 = call "PicoScope6000GetRapidBlockBulk_.vi"("error in"=w428, "handle in"=w433, "Rapid Block Acquisition Settings"=w422) -> ("Channel A Buffer"=w424:i16[][], "error out"=w429:errorcluster, "handle out"=w425:i16)  [unwired: 7 in, 3 out]
    n179 = Enqueue Element(queue=w435, element=w424, timeout in ms (-1)=-1, error in (no error)=w430) -> (queue out=w434:refnum<queue>, timed out?=w431:bool, error out=w427:errorcluster)
    n180 = Unbundle By Name(w427) -> ()  [unwired: 1 out]
    n181 = Or(x=w431, y="Stop") -> (x .or. y?=w426:bool)
  }
  n182 = while {
    tunnel: w85 -> [w478]
    tunnel: w84 -> [w475]
    tunnel: [w477] -> w81
    tunnel: [w476] -> w80
    tunnel: w41 -> [w458]
    shift-right: [w473] -> w64
    shift-left: w11 -> [w450]
    shift-right: [w449] -> w63
    shift-left: w68 -> [w472]
    shift-right: [w470] -> _
    shift-left: w10 -> [w469]
    shift-right: [w468] -> _
    shift-left: w44 -> [w467]
    shift-right: [w456] -> _
    shift-left: w41 -> [w459]
    shift-right: [w462] -> _
    shift-left: _ -> [w443]
    shift-right: [w465] -> w48
    shift-left: w49 -> [_]
    shift-right: [w461] -> _
    shift-left: 0 -> [w460]
    shift-right: [w443] -> _
    shift-left: _ -> [_]
    border: u32 0 ("millisecond timer value") -> [_]
    stop <- w474 stop-if-true
    # "队列数组应该是2048×5行30列的数组(行是采样的总的波形数，列\n是采样点数，值是桶探测值)"
    # "孙论文使用的\n进化算法，这\n里不使用"
    n183 = Tick Count (ms)() -> (millisecond timer value=w454:u32)
    n184 = feedback-in #5(w454) -> ()
    n185 = feedback #5() -> (w455:u32)
    n186 = case shown="假" "Evolutionary" {
      tunnel: "Patterns to display" -> [_ w570]
      tunnel: w459 -> [w560 w564]
      tunnel: w443 -> [_ w569]
      tunnel: w460 -> [w561 w565]
      tunnel: [w561 w568] -> w461
      tunnel: [w560 w567] -> w456
      tunnel: w458 -> [_ w563]
      frame False {
      }
      frame True {
        n187 = Not Equal?(x=w565, y=0) -> (x != y?=w562:bool)
        n188 = case shown="真" w562 {
          tunnel: w570 -> [_ w579]
          tunnel: w564 -> [_ w577]
          tunnel: w569 -> [_ w576]
          tunnel: [w571 w572] -> w567
          tunnel: w563 -> [w571 _]
          frame False {
          }
          frame True {
            n189 = local read "Resolution"() -> (w578:i32)
            n190 = call "Order_Signals_from2D_.vi"("Scoring\n Power"=2 ("Scoring\n Power"), "Resolution"=w578, "Signals"=w576, "Pattern Indices"=w577) -> ("Descsending Indexes"=w580:i32[])  [unwired: 1 out]
            n191 = Add(x="Adaptive Slider", y=0.01) -> (x+y=w573:dbl)
            n192 = call "Adaptive_Indices_.vi"("Patterns to Use"=w579, "Resolution"=w578, "Adaptive Slider"=w573, "Compressive Indices"=w580) -> ("LUT"=w572:i32[])  [unwired: 1 out]
          }
        }
        n193 = Increment(x=w565) -> (x+1=w568:i32)
      }
    }
    n194 = Subtract(x=w454, y=w455) -> (x-y=w453:u32)
    n195 = Divide(x=u32 1000, y=w453) -> (x/y=→"Update Rate (Hz)":dbl)
    n196 = local read "Pulses/Pattern"() -> (w466:i32)
    n197 = case shown="\"Slave - LUT\", 默认" "DMD Mode" {
      tunnel: w478 -> [w603 w627]
      tunnel: [w598 w621] -> w477
      tunnel: [w599 w620] -> w476
      tunnel: [w601 w619] -> w449
      tunnel: w475 -> [w602 w626]
      tunnel: w472 -> [w592 w625]
      tunnel: w458 -> [w585 w628]
      tunnel: w466 -> [w607 _]
      tunnel: w456 -> [w606 _]
      tunnel: "Patterns to display" -> [w597 _]
      tunnel: "Evolutionary" -> [w605 _]
      tunnel: [w588 w628] -> w463
      tunnel: "learned" -> [w583 _]
      frame "Slave - LUT", Default {
        n198 = Multiply(x=w597, y=u32 2) -> (x*y=w595:u32)
        n199 = local write "total patterns"(w595) -> ()
        n200 = Multiply(x=w595, y=w607) -> (x*y=w610:u32)
        n201 = Select(t=i32[] [0, 5, 2, 3, 32, 18, 11, 41, 1, 120, 68, 56, 43, 59, 200, 38, 6, 10, 96, 464, 216, 264, 192, 166, 14, 108, 60, 162, 165, 35, 69, 156, 104, 9, 144, 132, 199, 71, 848, 61, 143, 26, 196, 22, 768, 8, 816, 29, 1824, 46, 204, 992, 234, 62, 222, 189, 20, 39, 103, 124, 42, 50, 65, 207, 1040, 652, 185, 93, 239, 164, 161, 650, 368, 17, 644, 752, 111, 19, 584, 168, 766, 57, 24, 224, 203, 107, 45, 128, 236, 102, 21, 266, 115, 187, 864, 3360, 122, 176, 344, 608, 620, 163, 488, 648, 70, 101, 158, 545, 138, 728, 1004, 2568, 91, 227, 219, 540, 148, 340, 720, 398, 89, 1016, 560, 218, 40, 520, 1440, 33, 152, 3008, 2580, 384, 109, 237, 553, 167, 3200, 44, 616, 110, 100, 793, 15, 558, 131, 51, 261, 197, 929, 782, 3936, 432, 268, 123, 117, 409, 765, 751, 382, 175, 1002, 1029, 154, 924, 1044, 907, 923, 2565, 937, 814, 651, 998, 446, 328, 55, 534, 397, 30, 13, 854, 72, 503, 271, 255, 808, 942, 532, 790, 2584, 3148, 195, 2976, 217, 486, 136, 800, 452, 887, 632, 183, 614, 252, 34, 572, 618, 795, 2928, 3672, 772, 1628, 430, 367, 87, 853, 613, 4040, 990, 830, 533, 746, 528, 280, 1392, 2144, 1660, 2408, 349, 492, 3714, 3312, 813, 130, 388, 960, 841, 2136, 205, 1008, 3164, 749, 3280, 968, 2704, 724, 153, 741, 37, 738, 885, 211, 948, 220, 539, 2892, 470, 903, 3149, 3549, 338, 781, 339, 898, 3541, 79, 469, 653, 1776, 392, 835, 3960, 2773, 655, 917, 406, 1003, 519, 819, 645, 396, 457, 593, 435, 1001, 787, 902, 977, 3154, 771, 3948, 1356, 2528, 419, 997, 2412, 134, 225, 350, 4029, 2582, 226, 49, 617, 947, 1472, 629, 1592, 3392, 2336, 63, 86, 2832, 2256, 568, 4094, 391, 762, 472, 536, 1664, 121, 2870, 1340, 896, 803, 2861, 1376, 78, 2013, 429, 893, 2816, 362, 530, 381, 114, 3004, 249, 3472, 76, 582, 3196, 2844, 82, 2348, 514, 798, 870, 3864, 3727, 2424, 375, 1768, 3451, 428, 444, 3088, 53, 2468, 2140, 66, 1296, 3168, 544, 1548, 3966, 2485, 1618, 1550, 1007, 623, 3728, 4004, 232, 612, 722, 3917, 2692, 498, 2005, 807, 449, 734, 2416, 1692, 92, 3741, 3076, 1623, 2032, 882, 701, 727, 600, 2191, 2974, 656, 403, 812, 462, 387, 2178, 2493, 416, 2170, 2925, 3346, 2400, 209, 1468, 250, 411, 2518, 982, 1308, 523, 3304, 2194, 956, 1237, 863, 2392, 1388, 485, 2355, 792, 2410, 2948, 2328, 16, 1102, 1032, 3159, 581, 4021, 311, 3357, 1390, 975, 823, 4017, 99, 345, 2014, 3143, 547, 365, 3341, 463, 2591, 1223, 1612, 2766, 3142, 1705, 292, 343, 2566, 3642, 1988, 276, 1048, 1609, 2601, 3145, 155, 3608, 3676, 578, 3390, 3596, 3856, 4038, 706, 454, 3518, 3141, 1037, 177, 1288, 308, 3648, 2970, 2106, 3606, 1331, 2724, 1334, 1432, 1892, 3514, 1909, 3761, 3053, 901, 1230, 1429, 2876, 2293, 3086, 850, 141, 1951, 1822, 918, 1517, 1274, 1960, 414, 733, 1821, 3958, 723, 304, 3206, 659, 601, 3563, 36, 1170, 198, 3810, 1135, 3891, 3207, 3368, 3228, 1805, 337, 4056, 698, 1325, 2294, 1499, 660, 1527, 3003, 1321, 1738, 1184, 1140, 979, 2803, 717, 1342, 1065, 3244, 687, 2696, 314, 2204, 3445, 295, 1867, 1287, 1832, 4034, 3806, 3706, 2072, 2636, 2107, 935, 3679, 1854, 2420, 2435, 1708, 2112, 85, 890, 2842, 721, 987, 2474, 619, 2205, 2504, 3456, 3428, 2860, 2316, 919, 518, 3260, 932, 1513, 2959, 2213, 760, 2799, 753, 869, 1358, 442, 3494, 1758, 950, 3626, 2488, 3639, 669, 695, 1055, 3334, 810, 3524, 3403, 3913, 3804, 2324, 47, 564, 2711, 426, 1060, 1578, 2056, 1034, 1006, 1315, 3347, 3294, 1710, 394, 550, 354, 3967, 3686, 775, 1188, 1958, 2703, 4008, 571, 2932, 3956, 1894, 2183, 1899, 1810, 3063, 294, 3049, 3699, 3119, 3426, 25, 3187, 1295, 501, 2443, 3054, 2780, 2526, 3110, 1632, 985, 672, 2954, 3108, 1702, 2811, 1964, 2430, 3155, 1500, 2864, 3267, 2867, 3622, 1306, 2201, 2706, 3574, 2926, 3496, 3819, 2481, 2579, 630, 3435, 357, 484, 3752, 1243, 2896, 693, 2517, 949, 2270, 133, 2775, 1348, 1613, 2657, 2239, 1972, 3575, 3874, 1927, 1379, 833, 588, 1117, 688, 1791, 1920, 1035, 2514, 385, 2264, 2513, 1375, 1952, 1978, 2001, 301, 475, 1393, 1263, 1659, 702, 2917, 1586, 3749, 999, 1800, 1467, 3078, 3516, 1688, 1903, 3330, 2338, 2200, 3774, 778, 3041, 4052, 3327, 3825, 2548, 251, 291, 468, 838, 1030, 897, 3945, 322, 1772, 3404, 1136, 3234, 3431, 1246, 2628, 1103, 1371, 959, 2425, 1017, 3493, 2558, 3643, 3453, 180, 3128, 1196, 1354, 1973, 2555, 2768, 145, 2484, 2741, 774, 1977, 3241, 2197, 1051, 3421, 2515, 1407, 1244, 1605, 1703, 1652, 566, 3550, 3009, 351, 2824, 3268, 2633, 1523, 934, 1658, 606, 1732, 2384, 1792, 2857, 303, 1681, 666, 2853, 3746, 378, 3266, 4054, 2743, 2614, 2769, 3120, 1698, 300, 3530, 703, 2683, 208, 2330, 1458, 2576, 506, 1486, 1524, 1284, 984, 1162, 2402, 1104, 2405, 2924, 2995, 1275, 1121, 1430, 1537, 3272, 3118, 1286, 364, 2172, 3573, 1926, 2086, 1438, 1487, 1580, 1174, 2075, 3537, 4051, 852, 965, 1895, 1625, 319, 3245, 2119, 2538, 1619, 511, 1539, 604, 517, 675, 2918, 1347, 1679, 664, 267, 3036, 3286, 1855, 2749, 634, 1110, 2818, 3559, 2058, 2225, 3792, 3953, 2214, 2503, 352, 3594, 1213, 755, 1602, 1070, 1330, 3040, 3359, 1840, 1998, 1409, 3682, 333, 671, 1423, 3075, 3540, 2188, 3482, 1880, 3002, 1915, 3182, 1608, 1844, 731, 1741, 2873, 3045, 1547, 2356, 1946, 2698, 3438, 3816, 1980, 2943, 3510, 2965, 759, 2100, 2299, 142, 4041, 3709, 3013, 2097, 2145, 1337, 3449, 1164, 1815, 137, 2257, 2422, 2326, 3127, 3188, 3944, 2991, 2634, 2244, 1066, 3328, 3415, 3633, 3565, 2638, 1239, 859, 2911, 2268, 2777, 3767, 3174, 2573, 445, 1987, 2417, 2028, 3968, 3430, 1434, 4039, 1435, 3052, 2187, 479, 1558, 3894, 931, 2179, 3708, 3246, 1281, 1554, 1724, 2409, 2511, 2131, 1584, 1509, 2449, 221, 1881, 2520, 3219, 1381, 3906, 1606, 2418, 3015, 1750, 3269, 465, 1416, 1882, 3561, 2966, 685, 2463, 2810, 2296, 2878, 1759, 2462, 563, 2218, 3432, 77, 1590, 2008, 3342, 3239, 3201, 302, 3897, 2929, 2292, 127, 496, 3224, 595, 2459, 247, 289, 1370, 1795, 2403, 2646, 126, 3654, 1888, 3902, 2282, 1551, 2629, 3954, 2333, 3326, 2825, 2643, 401, 1479, 3122, 2608, 2900, 1647, 2265, 1300, 3409, 1154, 359, 433, 3202, 1078, 2478, 2585, 3802, 4091, 598, 1678, 320, 3189, 1464, 577, 3877, 589, 4062, 2372, 2057, 3687, 3423, 3566, 1441, 3090, 2687, 3668, 2763, 2670, 342, 1589, 2111, 1267, 3107, 1453, 1366, 3508, 3295, 3698, 1653, 3961, 3257, 3017, 3716, 2490, 1811, 2509, 3965, 936, 191, 2975, 880, 3680, 4084, 817, 2090, 1546, 2961, 1830, 3745, 1498, 1504, 1971, 633, 1294, 1224, 360, 2386, 2146, 2770, 318, 1859, 2129, 3520, 4014, 2897, 1530, 2457, 3829, 2828, 2640, 4047, 3490, 1473, 4031, 591, 3547, 1742, 2838, 2606, 920, 1823, 1400, 1731, 1645, 3920, 296, 4075, 3742, 535, 2421, 1413, 2942, 3492, 3434, 2489, 1251, 2276, 3485, 2501, 2830, 1917, 2994, 1671, 3014, 2171, 3882, 1412, 2625, 2388, 1885, 1582, 2054, 2062, 2690, 309, 2237, 1109, 1847, 4026, 3301, 3374, 3410, 2721, 1991, 1241, 1477, 1194, 3673, 1068, 2949, 2022, 1884, 1176, 1028, 1549, 3534, 4093, 2070, 3730, 425, 1496, 2423, 4010, 1119, 3436, 3638, 3740, 436, 2537, 2742, 3251, 2289, 363, 2709, 735, 1985, 412, 642, 3952, 3519, 2077, 2245, 1746, 3835, 3844, 3461, 1714, 1012, 1543, 2655, 3719, 2990, 1873, 2360, 3848, 2283, 1657, 2837, 1123, 1763, 2497, 1089, 3214, 2726, 3814, 2007, 1193, 1755, 3515, 3939, 459, 1418, 1399, 1817, 4024, 1257, 1361, 3546, 1715, 3647, 3715, 3990, 928, 1534, 3238, 473, 2891, 1013, 2556, 3985, 3023, 3553, 2250, 529, 4003, 1784, 1173, 2061, 1389, 1018, 2570, 1328, 2394, 3417, 1478, 2305, 3114, 269, 603, 1097, 298, 3056, 1529, 2487, 2231, 2505, 2135, 3860, 3366, 3832, 2989, 1207, 1874, 2547, 3760, 1394, 3697, 3137, 2447, 393, 1057, 3889, 4044, 3213, 88, 275, 3926, 1249, 1709, 2682, 1209, 1803, 408, 3998, 1206, 3535, 2571, 744, 3221, 2731, 2278, 2069, 1721, 1046, 2091, 4001, 3217, 945, 3418, 1984, 1019, 3318, 3780, 2805, 2125, 1783, 3980, 3419, 4079, 1635, 1093, 1433, 2586, 3775, 1607, 2820, 1098, 1428, 2677, 2060, 1782, 1493, 1545, 3645, 2154, 2455, 3000, 3243, 3710, 3766, 3930, 2506, 471, 1557, 3068, 3568, 2238, 4061, 955, 3805, 2102, 3803, 2232, 1465, 1075, 3656, 1175, 2672, 3337, 1794, 1583, 3564, 3395, 3773, 2779, 3813, 1976, 3319, 2729, 159, 1518, 2831, 1301, 3517, 828, 1957, 3290, 1343, 1218, 3125, 2390, 3034, 2373, 3759, 2914, 1491, 3667, 1215, 1825, 3898, 1310, 2450, 849, 3733, 1571, 4037, 1649, 1829, 1650, 3376, 2391, 2981, 4060, 3261, 3343, 3100, 3820, 1459, 2311, 3181, 84, 2964, 214, 1369, 3402, 1138, 1283, 2461, 3275, 3527, 3617, 2045, 2599, 2596, 2668, 3747, 3873, 1195, 3909, 2118, 491, 3971, 2691, 1670, 2230, 404, 2431, 3073, 1134, 1872, 1234, 2071, 1401, 1826, 2627, 2660, 1945, 3383, 2137, 2467, 1264, 1072, 537, 3552, 1074, 2442, 2699, 2841, 3999, 3943, 2997, 2757, 2113, 3950, 2133, 2224, 2471, 3281, 3842, 1163, 3763, 2735, 2945, 1959, 2151, 1561, 1492, 1764, 3962, 1651, 3924, 1905, 4030, 1690, 2242, 1085, 679, 2686, 2535, 1115, 691, 2764, 1211, 4066, 911, 2759, 769, 1850, 3250, 476, 3192, 4049, 1466, 1285, 3372, 609, 3875, 1200, 3979, 2772, 3881, 1526, 1185, 3837, 3411, 1385, 2658, 1058, 1532, 3681, 761, 3083, 2034, 3138, 3320, 258, 1568, 3895, 3158, 3307, 2475, 2315, 1111, 2127, 3197, 3047, 670, 962, 1455, 1043, 696, 1896, 2905, 639, 3042, 3997, 3593, 3332, 1317, 3636, 3499, 2168, 2472, 2274, 3536, 3161, 2645, 1447, 2143, 1120, 2353, 2221, 2921, 1520, 829, 2010, 3462, 3223, 3911, 2982, 3022, 2738, 2020, 1689, 1076, 3726, 3675, 3483, 3293, 3663, 3859, 1696, 2104, 3271, 1181, 2915, 2619, 3705, 1883, 3931, 1228, 2323, 2349, 1954, 1982, 2631, 1038, 3444, 3570, 2707, 3640, 2329, 1039, 2387, 2335, 1364, 843, 1836, 3033, 3385, 2260, 3351, 785, 3905, 3325, 3087, 431, 1335, 2371, 248, 1261, 565, 3391, 3556, 2228, 1449, 2395, 2563, 2017, 1125, 513, 2141, 3604, 2319, 2389, 1875, 147, 2039, 1146, 2280, 1454, 2404, 1912, 3750, 2840, 1205, 2577, 2624, 3441, 2543, 3215, 3712, 2139, 1639, 3309, 1788, 3487, 2734, 1216, 2817, 3193, 3464, 285, 1152, 826, 3598, 2153, 3603, 347, 2524, 2936, 2216, 1565, 2180, 2277, 2642, 3355, 1197, 2947, 3845, 2712, 1221, 2321, 2938, 3977, 1831, 3484, 3620, 2930, 1677, 2163, 3229, 2776, 2987, 3855, 1886, 583, 3694, 527, 2968, 3220, 1730, 3358, 1304, 1336, 3701, 585, 4023, 2266, 3811, 2219, 2393, 1666, 3377, 1183, 3448, 1841, 2893, 1282, 1227, 2248, 2637, 2604, 2068, 857, 2855, 1289, 369, 3082, 2087, 169, 3671, 2209, 736, 3232, 2813, 1516, 2241, 3893, 3588, 2291, 2758, 1171, 1834, 1656, 3946, 2656, 3869, 866, 2793, 1025, 1178, 3723, 3850, 3836, 3300, 2935, 1350, 316, 188, 1849, 1482, 2639, 1005, 3399, 1574, 2795, 2931, 1131, 1535, 2717, 1327, 2251, 3981, 3364, 1853, 3707, 2317, 2933, 1033, 1324, 2671, 2674, 3901, 2728, 855, 3928, 3507, 3353, 2273, 2025, 2676, 3058, 324, 3879, 2969, 1879, 2334, 3597, 3770, 1461, 2303, 2398, 3208, 3005, 1672, 2550, 2553, 2899, 1083, 1699, 2835, 3910, 3700, 851, 2051, 3887, 3489, 3059, 2081, 1198, 1497, 1852, 2689, 3095, 146, 2957, 3862, 2661, 2978, 2052, 1686, 2597, 4036, 1579, 3460, 3486, 2088, 3724, 3932, 681, 705, 2108, 497, 3665, 1424, 1599, 2243, 743, 3592, 3784, 3513, 2874, 3046, 2313, 3963, 1781, 3569, 2906, 3291, 2564, 28, 242, 260, 1250, 3080, 3129, 3336, 2952, 3957, 3629, 2130, 676, 2161, 3084, 1522, 2751, 490, 3801, 1054, 3776, 2836, 1233, 3370, 3793, 1889, 3211, 3439, 3892, 174, 1970, 2103, 3755, 1349, 2314, 2508, 2653, 2175, 3818, 2203, 1444, 2600, 1739, 2834, 3947, 2587, 2210, 3096, 708, 1167, 4048, 2602, 963, 1931, 1280, 3941, 2823, 1148, 2890, 3876, 2365, 3367, 3581, 3521, 1303, 2080, 3590, 3632, 3817, 2358, 4089, 1168, 3693, 1112, 3225, 2496, 3959, 1950, 1965, 2730, 958, 1106, 1225, 1560, 2414, 2641, 1151, 996, 1963, 3849, 2223, 3973, 2162, 3809, 3605, 2429, 451, 1460, 1415, 2345, 1130, 3616, 1417, 3361, 4090, 3624, 2539, 2174, 2846, 3247, 3912, 3505, 836, 1144, 3786, 1773, 2613, 2883, 1165, 3077, 230, 1355, 2882, 1450, 3711, 3475, 1662, 2525, 2233, 3557, 2033, 1838, 2357, 3781, 2885, 3512, 1887, 3649, 3276, 1081, 1769, 1357, 2158, 2259, 2845, 3867, 2575, 2138, 2498, 1983, 2325, 3562, 4053, 3506, 417, 3339, 2350, 2085, 2623, 4063, 4081, 914, 3458, 1127, 2368, 2651, 1801, 2722, 3035, 2647, 1141, 2886, 2263, 834, 2659, 3900, 3476, 1150, 1908, 1320, 74, 228, 1494, 2607, 2287, 3194, 2343, 1733, 3459, 3554, 3838, 3029, 2318, 3324, 2560, 3397, 509, 1309, 1814, 1307, 2454, 1566, 4011, 3094, 1638, 3621, 2157, 1687, 3400, 2733, 2937, 1949, 1298, 1540, 3509, 2029, 1095, 3830, 3690, 1665, 3139, 2165, 1419, 2369, 1994, 2066, 1266, 3027, 2685, 2716, 2298, 178, 3938, 2142, 3627, 3650, 1735, 1166, 1765, 2541, 3787, 2067, 1235, 2848, 2370, 1777, 4020, 3769, 3883, 2297, 1378, 2798, 489, 3975, 3543, 2094, 680, 1876, 2428, 1711, 1942, 1139, 2888, 1634, 1312, 2295, 3778, 2557, 1655, 1541, 3890, 1199, 3807, 2073, 3602, 2851, 3828, 2362, 3413, 3133, 3298, 1061, 3610, 986, 776, 3345, 3583, 2863, 4069, 3010, 1469, 2164, 2173, 3685, 4033, 1262, 1353, 2159, 2176, 1806, 3011, 3126, 2977, 839, 4073, 305, 895, 2783, 3313, 3866, 2822, 3661, 1937, 1614, 3989, 2346, 946, 307, 2745, 2267, 2150, 1346, 3050, 692, 1462, 1569, 1947, 556, 4055, 3674, 2434, 3655, 3316, 1367, 3851, 2666, 587, 3582, 1217, 3871, 2037, 1719, 611, 2916, 1862, 1092, 119, 1276, 2030, 1555, 395, 2719, 1107, 2688, 2789, 1754, 1071, 1940, 1685, 3350, 1981, 2839, 3914, 1622, 3481, 423, 281, 3695, 2236, 3113, 2581, 3669, 1490, 3623, 3424, 2049, 1299, 3986, 1910, 3109, 2397, 3595, 2611, 1155, 3822, 1643, 3771, 2519, 2301, 3853, 3135, 2385, 3843, 1124, 1231, 3001, 682, 1222, 3923, 3907, 551, 3933, 4042, 2275, 3833, 282, 2782, 3305, 3394, 2309, 2169, 2211, 3751, 3389, 1646, 3579, 73, 3454, 1925, 1726, 3463, 3951, 2247, 3729, 3840, 3978, 2043, 1302, 3847, 635, 3016, 4050, 1277, 2047, 3857, 2038, 1386, 1067, 2750, 1581, 1575, 2801, 2983, 3173, 1706, 2829, 1922, 961, 2521, 2352, 3544, 3779, 2381, 1948, 2262, 1273, 767, 3823, 2121, 3162, 3587, 1445, 2529, 4006, 3788, 2907, 270, 2621, 348, 3903, 879, 1704, 541, 2117, 3273, 2441, 1425, 1921, 3922, 2748, 1156, 2354, 95, 2031, 2374, 1916, 1153, 3112, 3502, 3043, 2697, 2337, 500, 607, 1256, 1437, 3491, 2495, 3190, 4074, 3070, 1955, 3227, 3274, 3578, 1869, 2426, 3198, 3571, 3691, 2255, 1684, 4068, 1953, 673, 994, 667, 1775, 1137, 2753, 3739, 1868, 3841, 1259, 2053, 1770, 658, 3178, 1941, 3865, 2304, 48, 371, 973, 3615, 1161, 1891, 718, 2041, 3858, 2723, 3988, 283, 1745, 2331, 3677, 2960, 3497, 3308, 1923, 1374, 686, 1914, 2673, 1084, 2979, 1966, 3995, 1691, 2797, 1939, 2713, 1694, 1064, 2923, 2470, 1377, 3748, 3115, 3235, 3955, 2540, 1047, 1785, 2439, 2220, 3226, 1725, 3826, 3136, 2185, 2593, 3721, 2958, 1809, 930, 1835, 665, 2415, 3772, 3101, 2004, 1397, 2019, 3240, 3344, 1890, 2980, 3754, 3365, 1431, 1564, 2300, 594, 2132, 2650, 2021, 2603, 3081, 1900, 1898, 297, 3085, 3479, 3405, 1202, 2050, 3369, 2327, 2269, 1252, 135, 1403, 1297, 1934, 3577, 2065, 4085, 2826, 2732, 2595, 299, 2095, 2341, 2662, 4027, 1191, 3737, 1505, 1943, 1069, 3666, 2026, 2675, 3495, 1475, 1096, 3097, 1999, 2227, 3210, 2920, 400, 2901, 3093, 1439, 1027, 3812, 3555, 1094, 2612, 2000, 1511, 3635, 1878, 3684, 2023, 2527, 1995, 1187, 2710, 1636, 1760, 3613, 3704, 1819, 2011, 3474, 3467, 2702, 3311, 1654, 3653, 1974, 3179, 2361, 3630, 317, 1833, 2206, 1902, 2096, 4070, 2554, 2884, 3186, 1717, 2654, 3531, 2059, 1740, 3393, 3331, 1338, 1536, 2854, 2110, 3249, 4015, 3322, 31, 2985, 1597, 3099, 1751, 2791, 2523, 1362, 3659, 2669, 3457, 4059, 3396, 2996, 1255, 913, 2074, 1796, 2339, 1767, 1050, 3795, 1384, 1226, 2913, 2009, 2193, 4007, 238, 2705, 1159, 2679, 3713, 2894, 3321, 105, 1877, 1938, 3362, 3105, 1913, 1837, 1090, 1865, 2084, 4045, 1845, 3644, 2452, 1313, 3265, 2444, 3420, 3839, 1747, 3204, 3983, 2532, 1637, 4019, 2785, 748, 1737, 3205, 2466, 1700, 346, 3030, 3422, 1442, 1471, 3117, 3545, 1828, 1210, 3277, 1572, 2502, 1100, 3306, 1073, 2701, 2016, 3425, 2413, 3177, 2347, 1145, 3994, 2078, 2963, 2445, 2271, 2212, 2407, 1099, 4083, 3878, 2644, 2872, 3757, 2788, 1979, 2105, 508, 441, 3471, 1820, 715, 2215, 1077, 2761, 3927, 3870, 783, 2198, 287, 1787, 1778, 2288, 2098, 3585, 1180, 1857, 624, 2592, 809, 3398, 2427, 3641, 579, 1932, 2064, 1293, 1661, 1091, 840, 2549, 1858, 2079, 81, 1712, 1332, 1682, 1443, 646, 1351, 3614, 3299, 1041, 3782, 2453, 1761, 1133, 3522, 1421, 905, 883, 2036, 2093, 75, 747, 1588, 1804, 3896, 1757, 1986, 2678, 3511, 2375, 2516, 3611, 3209, 3821, 1600, 2652, 3652, 448, 2919, 3796, 1485, 2063, 1594, 726, 3152, 1587, 1476, 1683, 1603, 2889, 2451, 2306, 3722, 3473, 1577, 3066, 1707, 2910, 1265, 3589, 561, 3102, 1059, 1593, 2809, 3852, 3091, 2561, 3764, 3789, 1673, 2754, 313, 3469, 3572, 1718, 2494, 3170, 1559, 3551, 2491, 2226, 1129, 2134, 2756, 2126, 2359, 3523, 2626, 2786, 116, 1693, 1591, 3028, 1160, 3815, 2076, 2253, 1753, 3150, 690, 2437, 784, 1521, 2999, 1147, 4058, 2787, 1179, 1373, 1253, 1446, 2546, 2812, 3287, 1451, 3195, 3185, 3191, 1631, 2583, 2833, 3765, 1101, 3303, 3231, 2941, 4032, 1236, 2377, 4000, 3798, 3609, 466, 3689, 2794, 957, 602, 1723, 2866, 3007, 2807, 3254, 615, 3144, 567, 2235, 2401, 2290, 3904, 1042, 1771, 4002, 2406, 3062, 2778, 3899, 3018, 4065, 2024, 386, 2973, 2363, 1611, 3183, 1756, 1023, 4018, 2665, 1269, 1601, 2806, 1633, 4057, 1113, 1319, 2258, 1339, 1744, 1189, 1116, 894, 1411, 1542, 662, 3060, 1383, 2545, 1169, 2166, 3121, 2865, 1553, 1182, 2465, 125, 3363, 1391, 3412, 2114, 3270, 1240, 2015, 2399, 2871, 4064, 306, 460, 875, 2123, 1563, 1474, 3762, 2082, 2739, 3915, 284, 1743, 976, 3558, 3591, 2879, 1956, 3607, 3664, 1305, 2700, 1268, 1839, 3799, 1667, 2499, 439, 1798, 818, 3222, 3089, 494, 657, 3340, 2115, 2986, 3285, 2747, 2376, 3039, 2815, 4035, 1208, 1314, 3600, 2632, 3279, 562, 2971, 2190, 3884, 2479, 2858, 2856, 3861, 2252, 1510, 1214, 3934, 1503, 332, 4092, 3548, 1669, 273, 3916, 1641, 2099, 1893, 2598, 796, 3151, 2411, 3106, 1481, 1045, 4012, 953, 2148, 467, 1596, 1827, 1624, 2819, 873, 754, 3414, 1247, 1480, 2378, 3465, 2469, 2364, 1919, 3233, 118, 1961, 2046, 1734, 2903, 3827, 1311, 2279, 2635, 1906, 1380, 3678, 1126, 1142, 2254, 1395, 3284, 3401, 3450, 3993, 3348, 3048, 3131, 542, 3477, 3381, 447, 683, 921, 2155, 1799, 1363, 1508, 427, 2746, 495, 2956, 2101, 3123, 3378, 4071, 610, 1668, 3601, 3991, 1080, 3255, 3725, 1063, 1774, 1483, 2902, 2737, 3379, 1203, 1556, 3628, 1368, 1816, 3032, 1365, 2664, 2714, 1232, 4025, 2234, 3111, 592, 377, 2018, 2366, 2367, 1866, 2027, 171, 995, 3153, 3743, 811, 4043, 3026, 569, 2340, 1105, 3657, 801, 3567, 2302, 1254, 2510, 3259, 3703, 2988, 2578, 3283, 1585, 3314, 580, 1122, 2594, 3868, 1897, 2382, 2934, 1729, 3297, 3175, 3753, 4080, 3785, 3282, 3863, 3791, 2588, 1642, 2953, 1514, 160, 2849, 293, 993, 2648, 3824, 2630, 2436, 3037, 1220, 699, 3386, 1212, 2951, 2680, 2993, 3065, 2887, 1842, 3808, 1329, 2530, 3831, 1396, 3854, 3480, 3949, 1118, 2736, 3532, 3584, 1507, 3940, 1398, 2821, 3375, 1290, 3919, 2800, 2109, 2620, 263, 3886, 2781, 1258, 3683, 3132, 1538, 1457, 356, 3935, 2035, 3972, 2483, 279, 2684, 1789, 3242, 1512, 1531, 888, 1762, 2725, 2663, 1452, 323, 3970, 1969, 1861, 1992, 1192, 3908, 374, 1062, 2569, 1495, 3625, 1177, 711, 2868, 241, 3382, 3576, 254, 2590, 4013, 2939, 847, 2615, 1848, 1087, 2922, 729, 3278, 2396, 202, 730, 3619, 2927, 1402, 3292, 1929, 2419, 370, 2284, 3637, 1748, 510, 3317, 678, 2286, 58, 420, 329, 262, 1279, 815, 1519, 3440, 3071, 2955, 1049, 622, 3218, 954, 2040, 3051, 832, 2480, 3427, 2605, 244, 2967, 970, 2616, 1573, 2881, 2380, 1132, 3289, 2610, 2383, 1422, 1793, 1567, 90, 1036, 1489, 1242, 3237, 1779, 1595, 3371, 3116, 312, 3203, 1749, 229, 991, 1387, 1818, 3734, 1627, 1996, 2877, 2246, 2222, 3356, 3452, 3756, 2149, 1640, 1962, 210, 2044, 3252, 3470, 3987, 740, 1871, 3373, 3992, 2771, 1219, 2307, 1157, 3169, 1172, 3315, 2124, 1501, 1149, 3783, 1697, 806, 23, 3929, 3407, 2342, 2667, 989, 3797, 1341, 2804, 455, 3736, 1904, 3885, 2217, 575, 2752, 3256, 2055, 1024, 3646, 1716, 3263, 3044, 1863, 3230, 290, 3074, 663, 797, 3031, 988, 951, 2522, 3503, 321, 2003, 2843, 1562, 4086, 1245, 713, 3072, 1528, 2229, 912, 555, 2177, 1291, 2322, 3248, 3447, 3019, 2249, 3442, 2458, 3323, 694, 700, 1701, 1918, 1626, 2207, 3236, 1736, 1292, 3612, 2542, 586, 1271, 422, 434, 1372, 1079, 3380, 3130, 2617, 2715, 2814, 3253, 1086, 3631, 1143, 278, 2559, 2092, 1935, 1323, 3199, 2718, 380, 80, 3012, 1846, 3021, 2083, 54, 3888, 1552, 2351, 2802, 725, 2618, 3599, 3964, 966, 1663, 2281, 157, 3539, 3067, 1088, 3768, 3542, 697, 758, 3171, 2912, 1617, 3777, 2694, 2156, 2762, 1930, 2167, 1414, 1186, 709, 605, 3732, 1790, 1463, 413, 904, 1797, 3172, 1576, 2531, 3006, 1695, 2790, 3800, 3662, 2998, 3147, 2875, 825, 668, 4076, 3408, 2681, 2784, 643, 981, 3500, 2850, 2944, 3758, 3925, 1114, 1630, 94, 2500, 272, 1382, 2332, 2320, 2909, 2895, 1502, 3651, 3103, 2122, 2562, 777, 925, 1780, 2827, 1870, 1720, 2261, 2859, 3302, 3618, 1420, 4067, 3580, 531, 2898, 3455, 341, 2507, 2477, 1108, 2482, 3670, 1408, 1975, 938, 969, 3310, 2536, 3388, 3429, 3937, 2446, 3134, 521, 3329, 3433, 3057, 3167, 4077, 974, 186, 674, 4022, 112, 1406, 2379, 1359, 2551, 886, 1082, 661, 1674, 1802, 4078, 1615, 716, 573, 1766, 3478, 2042, 3982, 2012, 3335, 1326, 3038, 1238, 3258, 327, 710, 3262, 2006, 315, 865, 487, 1426, 3942, 1616, 590, 1967, 1851, 1436, 3846, 286, 1470, 2649, 526, 3025, 2609, 3692, 2308, 1924, 3064, 1506, 1427, 1812, 881, 3790, 3834, 2534, 1843, 1405, 3586, 2182, 1026, 3163, 2622, 3446, 2904, 1352, 1675, 1448, 1278, 2862, 1270, 3996, 1629, 1020, 2147, 12, 1807, 3406, 190, 1933, 231, 2196, 3634, 3560, 2312, 2708, 3918, 334, 3969, 1907, 482, 2544, 2693, 3079, 654, 599, 274, 1333, 978, 538, 2192, 3166, 3498, 4072, 2847, 2774, 1533, 1201, 67, 3744, 1056, 707, 2492, 2120, 213, 4082, 2760, 2116, 2473, 844, 4, 1722, 3160, 3354, 1128, 4009, 474, 2755, 916, 3124, 3216, 906, 1727, 2152, 83, 549, 1570, 845, 3092, 2727, 1856, 570, 4005, 3718, 861, 3974, 4028, 2533, 1786, 493, 1316, 3660, 2796, 640, 2189, 3055, 4087, 805, 194, 3338, 399, 2486, 1410, 1272, 1713, 113, 2344, 3720, 1610, 150, 856, 1345, 2433, 3921, 967, 2272, 481, 788, 1808, 2440, 3098, 1318, 3387, 2310, 677, 597, 3416, 223, 3069, 2984, 2476, 971, 2186, 3501, 390, 1021, 2208, 3333, 2089, 2285, 543, 2962, 3658, 2720, 1260, 1911, 2695, 980, 1620, 799, 2950, 1644, 3528, 3529, 1322, 3702, 548, 636, 1484, 1190, 52, 2240, 201, 2744, 3212, 596, 4046, 3437, 335, 2792, 424, 3526, 1009, 628, 1014, 1404, 625, 1015, 2002, 2869, 1456, 3146, 2740, 862, 732, 1525, 3165, 1360, 770, 310, 507, 546, 2202, 3738, 3443, 1968, 574, 846, 1928, 689, 505, 2464, 418, 253, 2574, 1515, 1813, 1993, 170, 867, 2160, 1936, 2438, 3794, 421, 277, 461, 714, 172, 3538, 2946, 2908, 483, 325, 3984, 2552, 184, 1997, 2972, 831, 149, 3872, 215, 1544, 820, 27, 559, 780, 802, 1648, 983, 2852, 3349, 3264, 940, 1621, 212, 456, 440, 779, 2767, 910, 98, 1344, 1248, 1944, 2432, 326, 1901, 499, 502, 361, 1031, 1204, 2589, 3061, 3468, 3184, 366, 233, 173, 3352, 1990, 512, 1598, 129, 719, 265, 878, 649, 3735, 106, 3731, 246, 97, 927, 2512, 1158, 3688, 2992, 259, 871, 288, 4016, 182, 450, 791, 892, 824, 3384, 389, 2199, 922, 684, 884, 757, 415, 889, 3104, 3180, 256, 2460, 1860, 1000, 576, 750, 1488, 477, 453, 621, 3157, 3140, 827, 794, 525, 355, 939, 3525, 3880, 3504, 3466, 376, 627, 952, 554, 2940, 1680, 2880, 804, 1011, 480, 1676, 2048, 353, 943, 891, 933, 2448, 712, 1229, 193, 915, 745, 257, 336, 868, 786, 552, 1989, 1728, 358, 2456, 3020, 637, 3296, 860, 181, 3176, 515, 516, 1010, 2184, 557, 405, 756, 379, 626, 151, 139, 458, 877, 4088, 899, 773, 941, 383, 372, 478, 1864, 763, 245, 243, 837, 2128, 407, 789, 3717, 2572, 638, 2195, 140, 2808, 858, 206, 438, 737, 872, 964, 7, 3024, 821, 908, 330, 235, 704, 443, 822, 3696, 876, 373, 3533, 2567, 900, 926, 641, 3156, 764, 3288, 437, 944, 742, 240, 2181, 1604, 909, 1752, 64, 1053, 2765, 522, 647, 972, 504, 631, 874, 179, 842, 739, 331, 1052, 1022, 524, 410, 402, 3488, 3976, 4095] ("Array"), s=w583, f=w585) -> (s? t:f=w584:i32[])
        n202 = Multiply(x=w610, y="Additional Data") -> (x*y=w608:dbl)
        n203 = To Unsigned Long Integer(number=w608) -> ()  [unwired: 1 out]
        n204 = Array Subset(array=w584, index=0, length=w597) -> (w600:i32[])
        n205 = Select(t=w606, s=w605, f=w600) -> (s? t:f=w588:i32[])
        n206 = Array Size(array=w588) -> (size(s)=w594:i32)
        n207 = case shown="真" TRUE ("Sync Frame") {
          tunnel: w588 -> [w613 w615]
          tunnel: [w613 w614] -> w587
          frame False {
          }
          frame True {
            n208 = Multiply(x=w615, y=2) -> (x*y=w617:i32[])
            n209 = Increment(x=w617) -> (x+1=w616:i32[])
            n210 = Interleave 1D Arrays(w617, w616) -> (w614:i32[])
          }
        }
        n211 = Decrement(x=w594) -> (x-1=w593:i32)
        n212 = flat-sequence {
          tunnel: [w612] -> w591
          tunnel: w592 -> [w612]
          frame #0 {
          }
        }
        n213 = Replace Array Subset(array=w588, new element=0 ("new element/subarray"), index=w593) -> ()  [unwired: 1 out]
        n214 = Build Array (concatenate)(w587, 1 ("new element/subarray")) -> (w586:i32[])
        n215 = call "Large_LUT_Mode_Slave_flash_.vi"("error in (no error)"=w591, "SequenceId"=w602, "DeviceIdPtr in"=w603, "LUT"=w586) -> ("error out"=w601:errorcluster, "SequenceId Out"=w599:u32, "DeviceId Out"=w598:u32)  [unwired: 5 in]
      }
      frame "Slave - All Patterns" {
        # "dmd显示之前\n加载的pattern"
        # "没用"
        # "FLUT没用"
        n216 = local read "total patterns"() -> (w630:i32)
        n217 = Decrement(x=w630) -> (x-1=w629:i32)
        n218 = call "ALP_FLUT_Mode_None_.vi"("error in (no error)"=w625, "SequenceId in"=w626, "DeviceId in"=w627) -> ("error out"=w624:errorcluster, "SequenceId out"=w623:u32, "DeviceId out"=w622:u32)  [unwired: 6 in]
        n219 = call "ALP_Sub_Pattern_.vi"("Last Frame"=w629, "First Frame"=0, "error in (no error)"=w624, "Repetitions"=0, "SequenceId in"=w623, "DeviceIdPtr in"=w622) -> ("error out"=w635:errorcluster, "SequenceId out"=w631:u32, "DeviceId"=w636:u32)  [unwired: 3 in]
        n220 = flat-sequence {
          tunnel: w635 -> [w637]
          tunnel: [w637] -> w634
          frame #0 {
            n221 = Wait (ms)(milliseconds to wait="ms to wait") -> ()  [unwired: 1 out]
          }
        }
        n222 = call "start_DLP_repetitions.vi"("error in (no error)"=w634, "SequenceId"=w631, "DeviceId"=w636) -> ("error out"=w619:errorcluster, "SequenceId Out"=w620:u32, "DeviceId Out"=w621:u32)  [unwired: 6 in]
      }
    }
    n223 = Get Queue Status(queue=w450, return elements? (F)=TRUE, error in (no error)=w449) -> (queue out=w448:refnum<queue>, error out=w447:errorcluster, # elements in queue=→"# elements 2":i32)  [unwired: 5 out]
    n224 = Dequeue Element(queue=w448, timeout in ms (-1)=-1, error in (no error)=w447) -> (queue out=w473:refnum<queue>, element=w438:i16[][], error out=w465:errorcluster)  [unwired: 1 out]
    n225 = for {
      tunnel: w438 -> [w559] mode=indexing
      tunnel: [w558] -> w439 mode=indexing
      workers-P: _ -> [_]
      # "对队列数组\n每行求均值"
      n226 = call-poly <vilib>:"Mean.vi"("X"=w559) -> ("mean"=w558:dbl)  [unwired: 1 out]
    }
    "?" <- w439
    n227 = Array Size(array=w438) -> (size(s)=w437:i32[])
    n228 = case shown="真" TRUE {
      tunnel: [w481 w522] -> w470
      tunnel: w469 -> [w481 w521]
      tunnel: [w480 w520] -> w468
      tunnel: w467 -> [w480 w519]
      tunnel: w463 -> [_ w489]
      tunnel: [w479 w515] -> w462
      tunnel: w439 -> [_ w495]
      tunnel: w438 -> [_ w493]
      tunnel: "Evolutionary" -> [_ w492]
      tunnel: w443 -> [w479 _]
      tunnel: "learned" -> [_ w490]
      tunnel: w437 -> [_ w484]
      frame False {
      }
      frame True {
        # "4"
        # "2048"
        # "转置回来"
        # "将板卡采集的原始数据队列(蓝)\n经过求平均和正负hadamard减\n的操作后得到一个30*1024数组\n送到一个由处理后探测值数列、\nhadamard矩阵、LUT(不用)组成\n的cropped signals队列(粉)"
        # "对每行求平均，获得\n每个像素点对应的\n30个探测值的平均值"
        # "选择一行显示一个波形的30个采样值，\n两张图横坐标一个是采样数，一个是时间(ns)"
        # "转置"
        # "再求均值得到\n数组所有值的均值"
        # "得到30*1024的数组，每行对应一个\nhadamard pattern的探测值，可以\n恢复出一幅32*32的图"
        # "从前面输出的某一行\n开始共截取2048*4行的数组"
        # "对截取后的2048*4行30列数组每四行拿出来对列求平均，\n使得每一行对应一张pattern所获得波形的采样值，得到\n行数/4=2048，列数30的数组"
        n229 = Or(x=w490, y=w492) -> (x .or. y?=w491:bool)
        n230 = call-poly <vilib>:"Mean.vi"("X"=w495) -> ("mean"=w502:dbl)  [unwired: 1 out]
        n231 = Array Size(array=w493) -> (size(s)=w504:i32[])
        n232 = while {
          tunnel: w493 -> [w527] mode=indexing
          tunnel: [w533] -> w483
          tunnel: w502 -> [w526]
          i -> [w533]
          stop <- w529 stop-if-true
          # "输出：数组从0行开始直到一行(行数＜2001)的\n最大值大于等于数组均值的两倍，输出这一行\n的行数或者输出2001"
          n233 = Array Max & Min(array=w527) -> (max value=w528:i16)  [unwired: 3 out]
          n234 = Multiply(x=w526, y=2.0) -> (x*y=w534:dbl)
          n235 = Less?(x=w534, y=w528) -> (x < y?=w530:bool)
          n236 = Less?(x=2000, y=w533) -> (x < y?=w531:bool)
          n237 = Or(x=w530, y=w531) -> (x .or. y?=w529:bool)
        }
        n238 = Index Array(array=w504, index=1) -> (element=w482:i32)
        n239 = local read "Pulses/Pattern"() -> (w500:i32)
        n240 = local read "total patterns"() -> (w501:i32)
        n241 = Multiply(x=w501, y=w500) -> (x*y=w499:i32)
        n242 = Array Subset(array=w493, index (row)=w483, length (row)=w499, index (col)=0 ("index"), length (col)=w482) -> (w505:i16[][])
        n243 = local read "Pulses/Pattern"() -> (w498:i32)
        n244 = Array Size(array=w505) -> (size(s)=w512:i32[])
        n245 = Index Array(array=w512, index #1=0 ("index"), index #2=1 ("index")) -> (element #1=w508:i32, element #2=w507:i32)
        n246 = Divide(x=w508, y=w498) -> (x/y=w509:dbl)
        n247 = for {
          N: w509 -> [_]
          tunnel: w505 -> [w551]
          tunnel: w507 -> [w550]
          tunnel: [w544] -> w496 mode=indexing
          tunnel: w498 -> [w545]
          i -> [w548]
          # "求平均(有一个过滤过程)"
          n248 = Multiply(x=w545, y=w548) -> (x*y=w547:i32)
          n249 = Array Subset(array=w551, index (row)=w547, length (row)=w545, index (col)=0 ("index"), length (col)=w550) -> (w546:i16[][])
          n250 = call "Oddwave Filter_.vi"("Wave Array Input"=w546) -> ("Averaged Wave Output"=w544:dbl[])  [unwired: 8 in, 1 out]
        }
        n251 = Transpose 2D Array(2D array=w496) -> (transposed array=w497:dbl[][])
        n252 = for {
          tunnel: w497 -> [w541] mode=indexing
          tunnel: [w536] -> w494 mode=indexing
          workers-P: _ -> [_]
          # "末位置0？"
          # "对正负hadamard pattern\n对应的桶探测值求差"
          n253 = Decimate 1D Array(w541) -> (w543:dbl[], w542:dbl[])
          n254 = Subtract(x=w543, y=w542) -> (x-y=w537:dbl[])
          n255 = Array Size(array=w537) -> (size(s)=w540:i32)
          n256 = Decrement(x=w540) -> (x-1=w539:i32)
          n257 = Replace Array Subset(array=w537, new element=0 ("new element/subarray"), index=w539) -> (w536:dbl[])
        }
        n258 = local read "Hadamards"() -> (w518:bool[][])
        n259 = Transpose 2D Array(2D array=w494) -> (transposed array=w513:dbl[][])
        n260 = Index Array(array=w513, index (row)="index (row)") -> (element=w485:dbl[])  [unwired: 1 in]
        "?" <- w485
        n261 = case shown="假" w491 {
          tunnel: w489 -> [_ w557]
          tunnel: w518 -> [w554 w556]
          tunnel: [w554 w555] -> w516
          frame False {
          }
          frame True {
            n262 = call "Index_patterns_.vi"("LUT"=w557, "All Patterns in"=w556) -> ("All Patterns out"=w555:bool[][])
          }
        }
        n263 = for {
          tunnel: w513 -> [w552] mode=indexing
          tunnel: [w553] -> w488 mode=indexing
          workers-P: _ -> [_]
          n264 = call-poly <vilib>:"Mean.vi"("X"=w552) -> ("mean"=w553:dbl)  [unwired: 1 out]
        }
        "?" <- w488
        n265 = for {
          tunnel: [w523] -> w487 mode=indexing
          tunnel: w485 -> [_] mode=indexing
          i -> [w524]
          n266 = Multiply(x=0.4, y=w524) -> (x*y=w523:dbl)
        }
        n267 = Bundle(w494, "All Patterns out"=w516, "LUT"=w489) -> (w517:T8)  [unwired: 1 in]
        n268 = Bundle(w487, w485) -> (→"pattern temporal signal":cluster{dbl[], dbl[]})  [unwired: 1 in]
        n269 = Build Array(w488) -> (w515:dbl[][])
        n270 = Enqueue Element(queue=w521, element=w517, error in (no error)=w519) -> (queue out=w522:refnum<queue>, error out=w520:errorcluster)  [unwired: 1 in, 1 out]
        "数组" <- w484
      }
    }
    n271 = call "Check Data_.vi"("Mean Prefiltered Signals"=w439) -> ("similar"=→"OK?":bool)  [unwired: 10 in]
    n272 = local read "Stop"() -> (w474:bool)
  }
  n273 = call "PicoScope6000Close.vi"("handle"=w69) -> ()
  n274 = Merge Errors(w70) -> (w71:errorcluster)
  n275 = call <vilib>:"Simple Error Handler.vi"("error in (no error)"=w71) -> ()  [unwired: 4 in, 5 out]
  n276 = Flush Queue(queue=w61, error in (no error)=w50) -> ()  [unwired: 3 out]
  n277 = Flush Queue(queue=w33, error in (no error)=w32) -> ()  [unwired: 3 out]
  n278 = Flush Queue(queue=w34, error in (no error)=w32) -> ()  [unwired: 3 out]
  n279 = Flush Queue(queue=w64, error in (no error)=w48) -> ()  [unwired: 3 out]
  n280 = call "stop_DLP_.vi"("error in (no error)"=w63, "SequenceId"=w80, "DeviceId"=w81) -> ("error out"=w79:errorcluster, "SequenceId Out"=w78:u32, "DeviceId Out"=w77:u32)  [unwired: 6 in]
  n281 = call "close_DLP_.vi"("error in (no error)"=w79, "SequenceId"=w78, "DeviceId"=w77) -> ("error out"=w83:errorcluster)  [unwired: 8 in]
  n282 = call <vilib>:"Simple Error Handler.vi"("error in (no error)"=w83) -> ()  [unwired: 4 in, 5 out]
